vi "A170316-11_Auto - 副本.vi"() -> ()   [LabVIEW 2020]
uses:
  2e0b5f5e-2208-4490-a798-25a802626be8.vi
  Global_Variable/A170316-11.vi
  Global_Variable/Global.vi
  Database/Global1.vi
  <vilib>/addons/database/Connection.llb/DB Tools Open Connec (String).vi
  <vilib>/regexp/Match Regular Expression.xnode
  <vilib>/addons/database/NI_Database_API.lvlib
panel:
  out "请拾取O型圈":bool
  out "请拾取弹簧":bool
  in  "控制器支架":T1(ring)
  in  "ECU步骤":T2(ring)
  in  "电机步骤":T3(ring)
  out "产品型号":string
  in  "更换产品":refnum<vi>
  in  "前序OK？_ECU":string
  in  "前序OK？":string
  in  "Process":string[](array[string])
  in  "Code":string[](array[string])
  in  "User":string[](array[string])
  in  "Result":string[](array[string])
  in  "Device":string[](array[string])
  out "安装支架螺栓4拧紧确认":bool
  in  "STEP2":string
  in  "STEP1":string
  out "控制器安装螺栓3拧紧确认":bool
  out "电机安装螺栓3扭矩确认":bool
  out "控制器支架螺栓5拧紧确认":bool
  out "安装扎带并取走工件":bool
  out "涂色标":bool
  out "按启动按钮拍照确认":bool
  out "电机安装螺栓2扭矩确认":bool
  out "电机安装螺栓1扭矩确认":bool
  out "安装支架涂色标":bool
  out "控制器安装螺栓2拧紧确认":bool
  out "控制器安装螺栓1拧紧确认":bool
  out "安装支架螺栓2拧紧确认":bool
  out "安装弹性垫圈弹簧并按启动拍照":bool
  out "安装支架螺栓1拧紧确认":bool
  out "控制器支架涂色标":bool
  out "控制器支架螺栓4拧紧确认":bool
  out "控制器支架螺栓3拧紧确认":bool
  out "控制器支架螺栓2拧紧确认":bool
  out "控制器支架螺栓1拧紧确认":bool
  out "安装支架螺栓3拧紧确认":bool
  in  "更换布局":string
  out "安装扎带和线卡并取走工件":bool
  out "安装支架扎带安装":bool
  out "安装支架线卡扎带安装":bool
  out "控制器支架安装线卡扎带":bool
  out "磨合次数":i32
  in  "判定结果":bool[][](array[boolean])=[[TRUE]]
  in  "STEP3":string
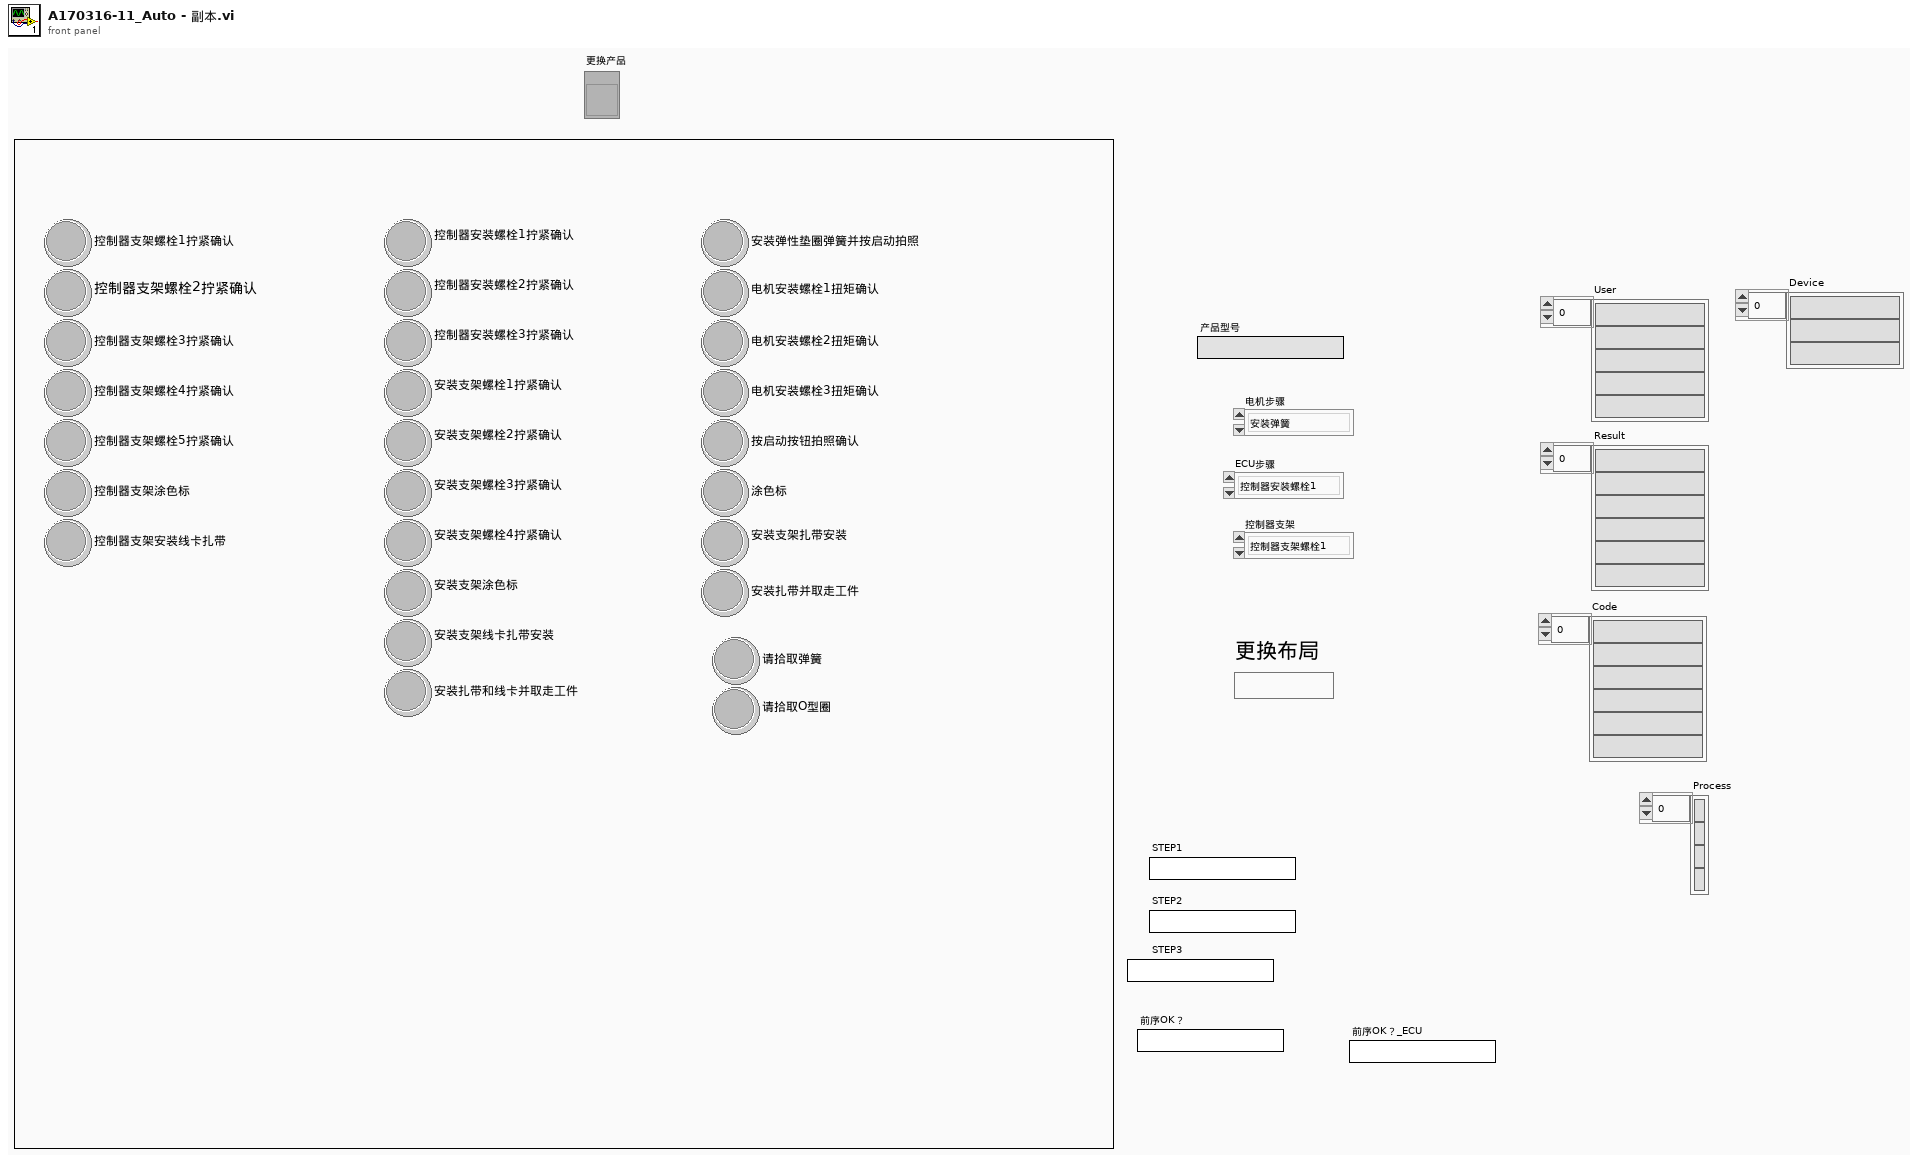
[diagram p1: front panel]
types:
  T1 = enum16{"控制器支架螺栓1", "控制器支架螺栓2", "控制器支架螺栓3", "控制器支架螺栓4", "控制器支架螺栓5", "涂色标", "安装线卡轧带", "完成"}
  T2 = enum16{"控制器安装螺栓1", "控制器安装螺栓2", "控制器安装螺栓3", "安装支架螺栓1", "安装支架螺栓2", "安装支架螺栓3", "安装支架螺栓4", "涂色标", "安装线卡轧带", "取走工件", "完成"}
  T3 = enum16{"安装弹簧", "安装O型圈", "安装弹性垫圈", "电机螺栓1", "电机螺栓2", "电机螺栓3", "电机拍照", "涂色标", "装轧带", "取走工件", "完成"}
  T4 = cluster{i64, i64, i64, "电机工位生产结果":string, "result string":string}
  T5 = cluster{i64, i64, i64, "电机工位生产结果":string, "result string":string}[]
  T6 = typedef "NI_Database_API.lvlib/Conn ObjectReference.ctl" = refnum<k1>
  T7 = cluster{"电机工位生产结果":string, "result string":string}
  T8 = cluster{i64, i64, i64, "ECU工位生产结果":string, "result string":string}
  T9 = cluster{i64, i64, i64, "ECU工位生产结果":string, "result string":string}[]
  T10 = cluster{"ECU工位生产结果":string, "result string":string}
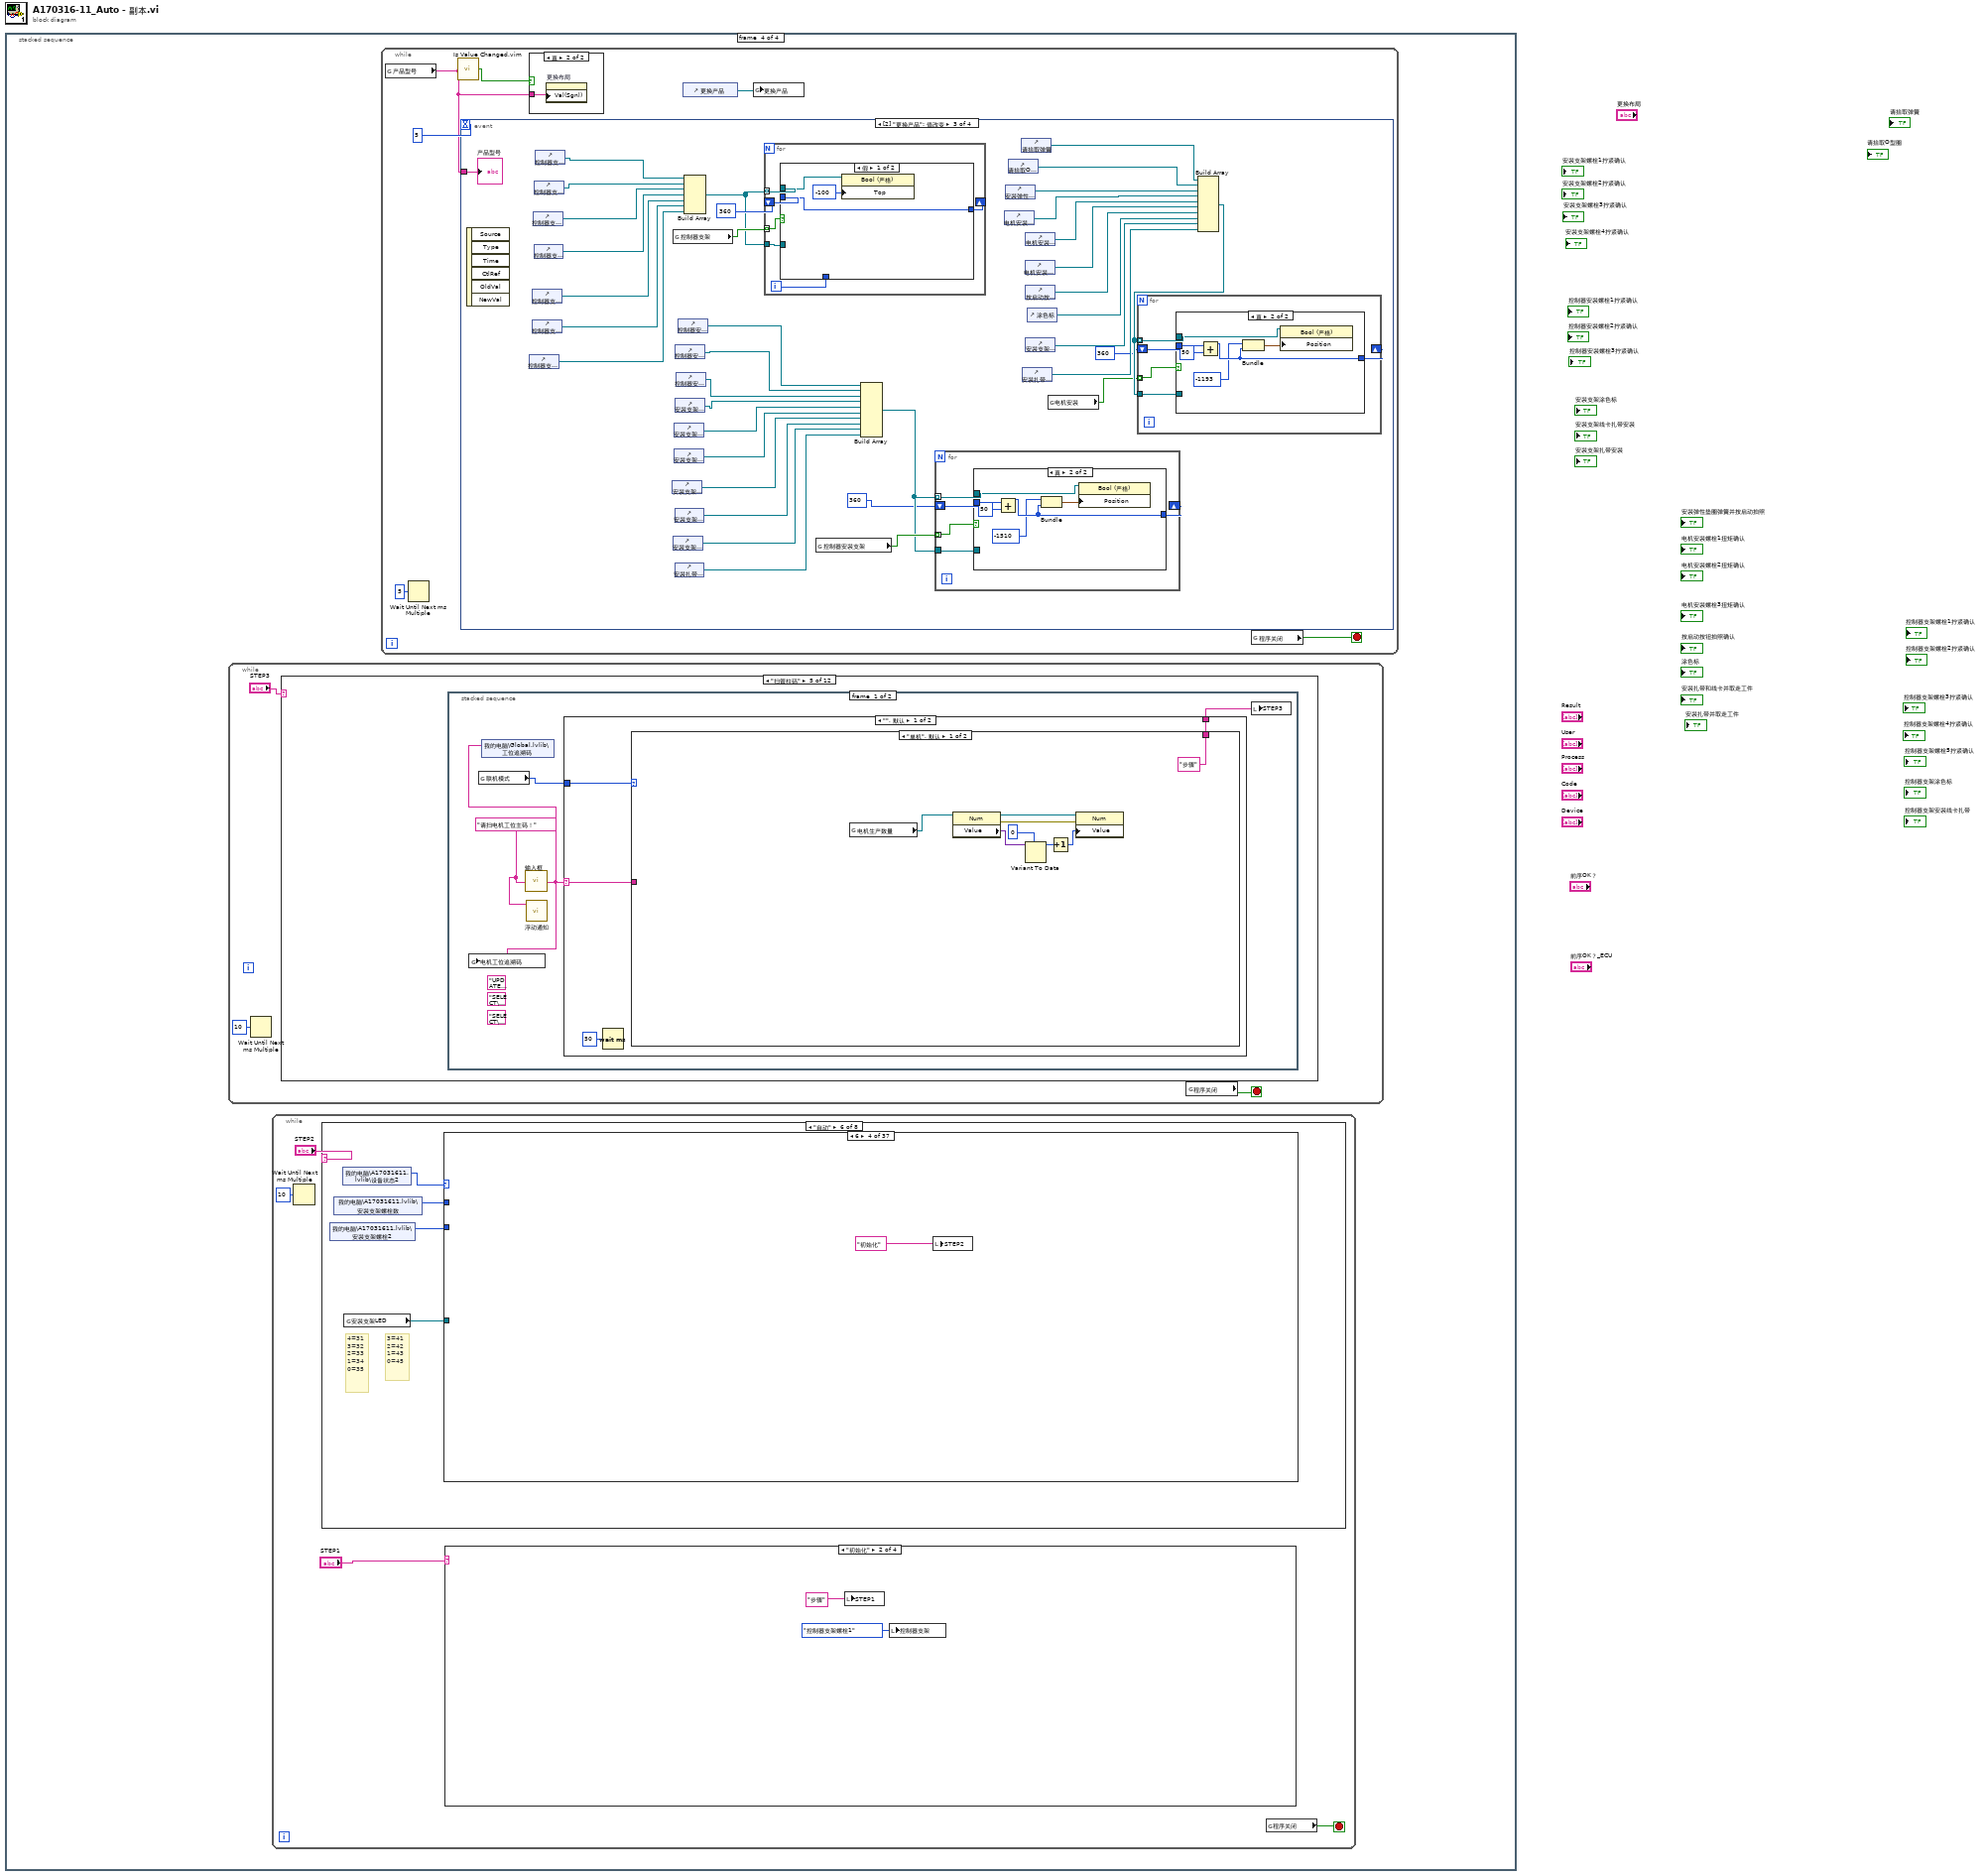
[diagram p0: block diagram]
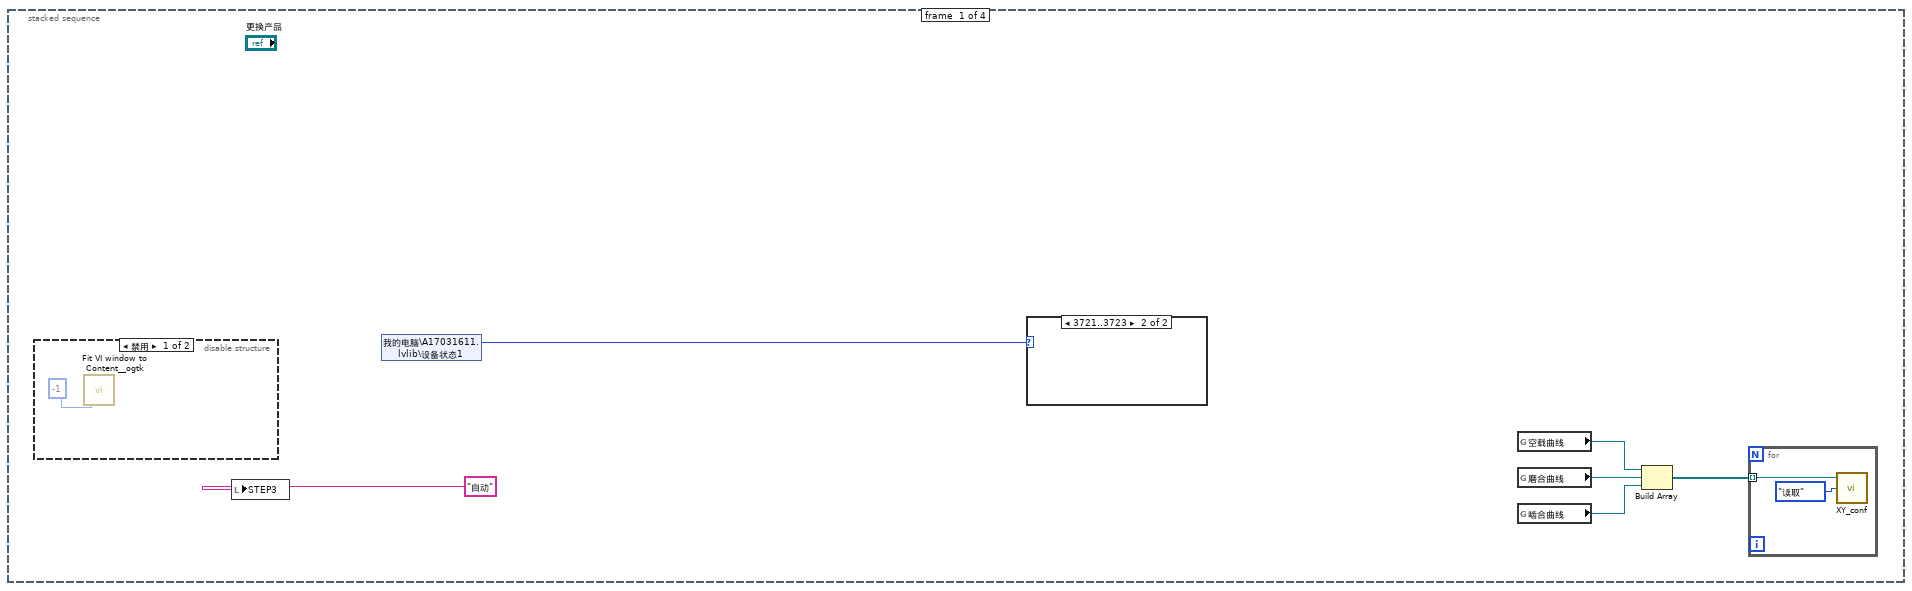
[diagram p2: hidden frame]
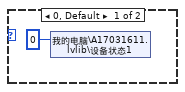
[diagram p4: hidden frame]
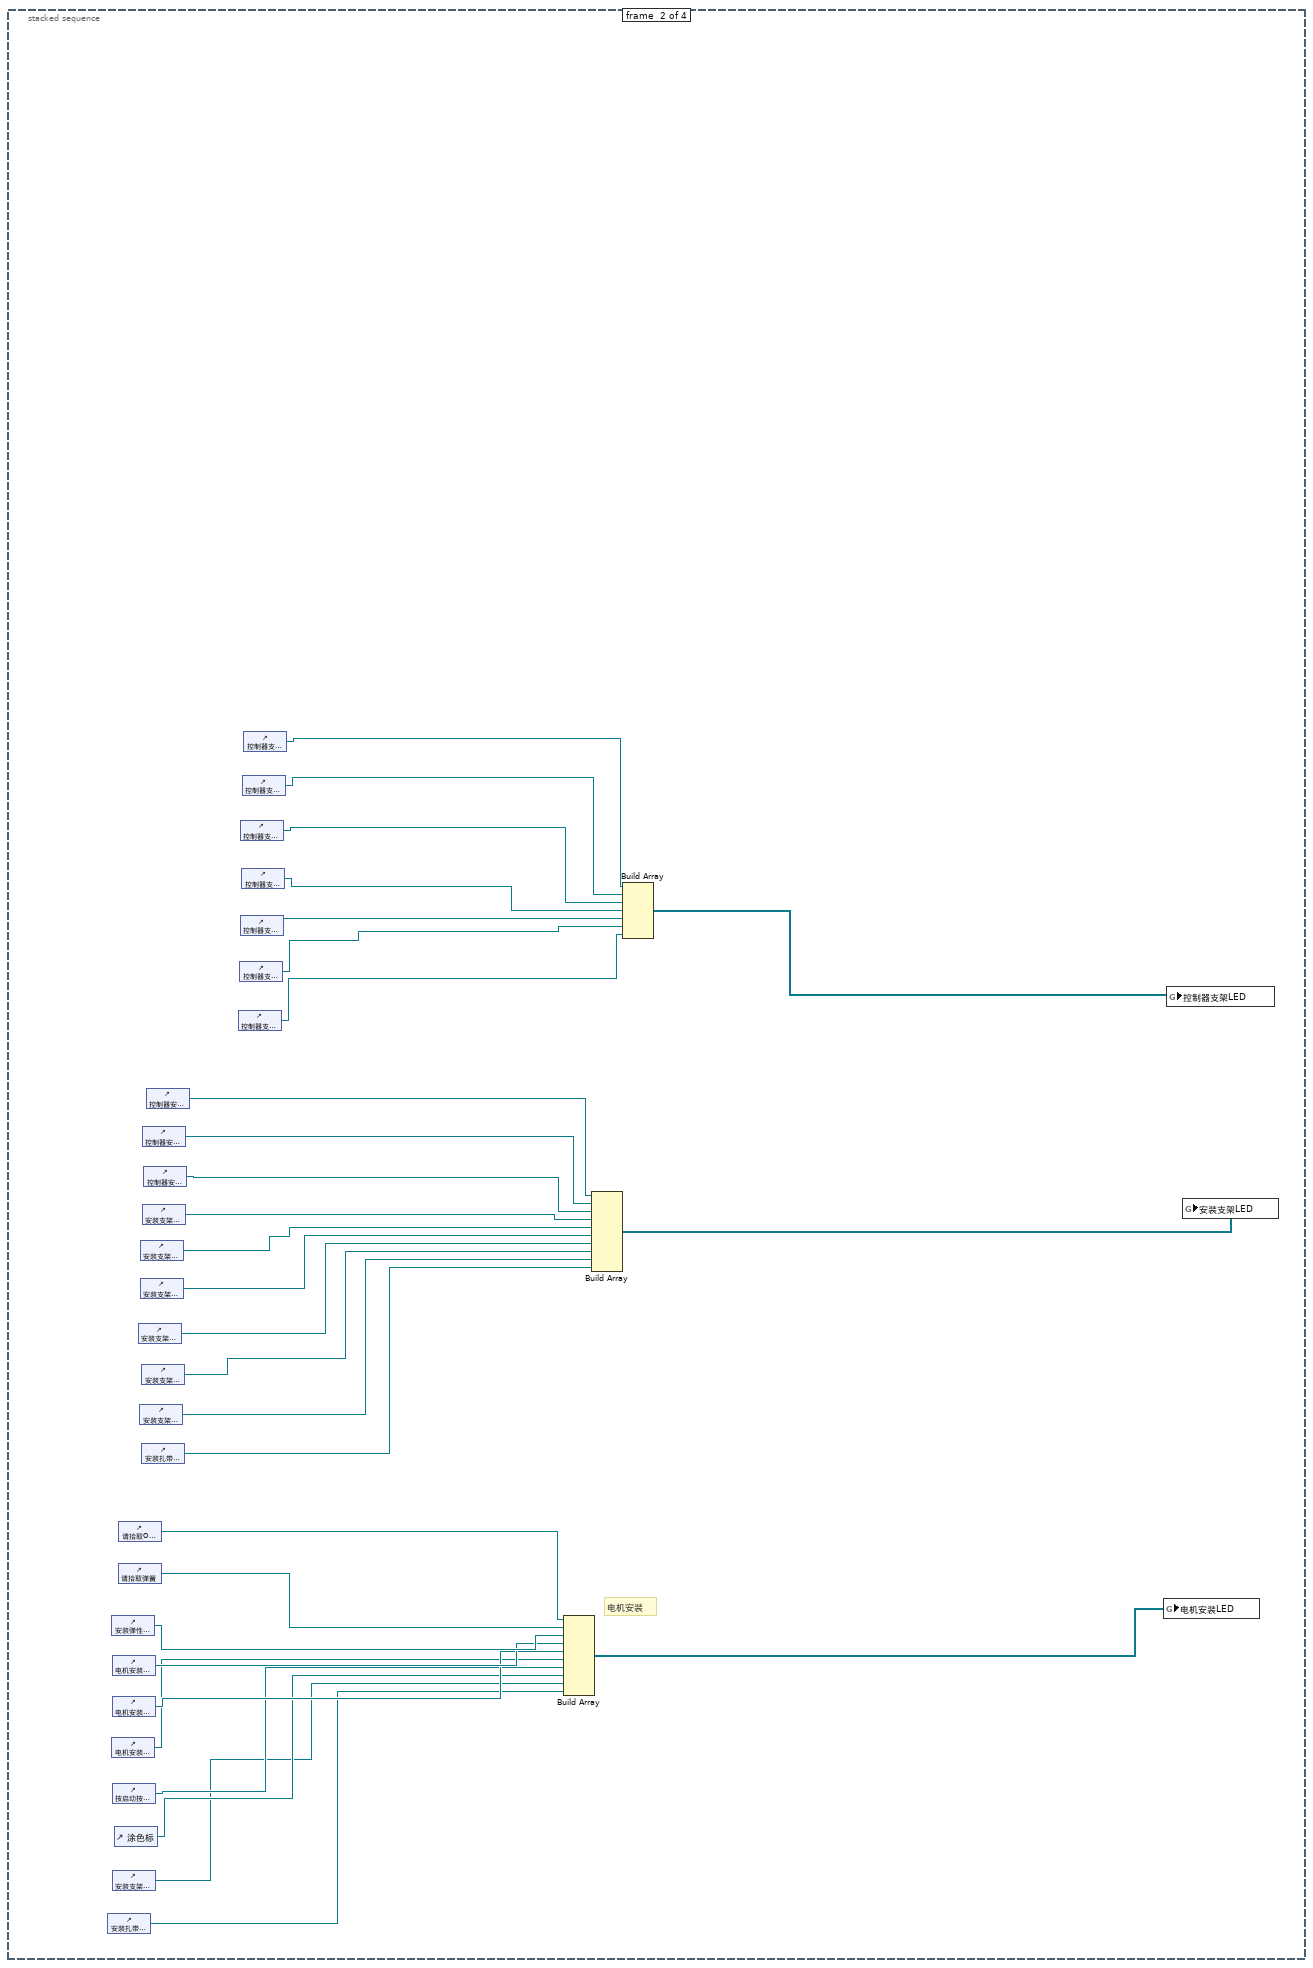
[diagram p5: hidden frame]
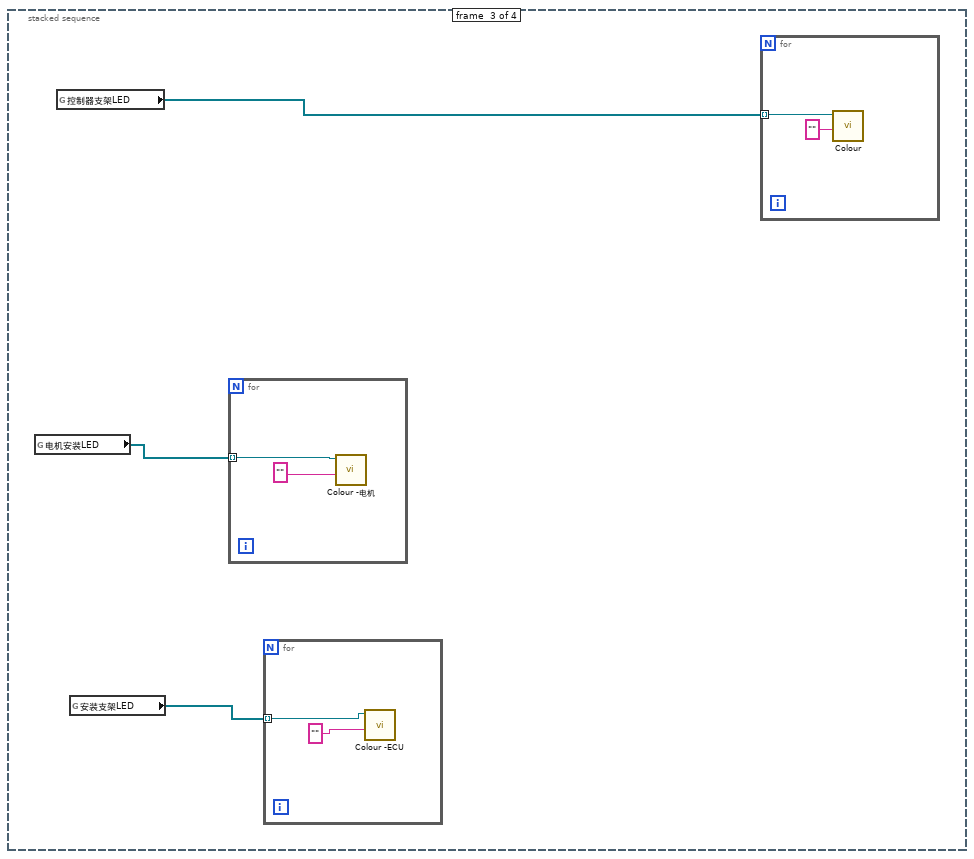
[diagram p6: hidden frame]
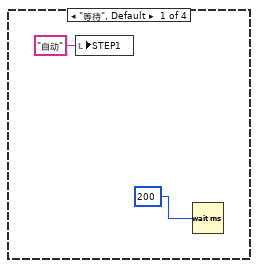
[diagram p7: hidden frame]
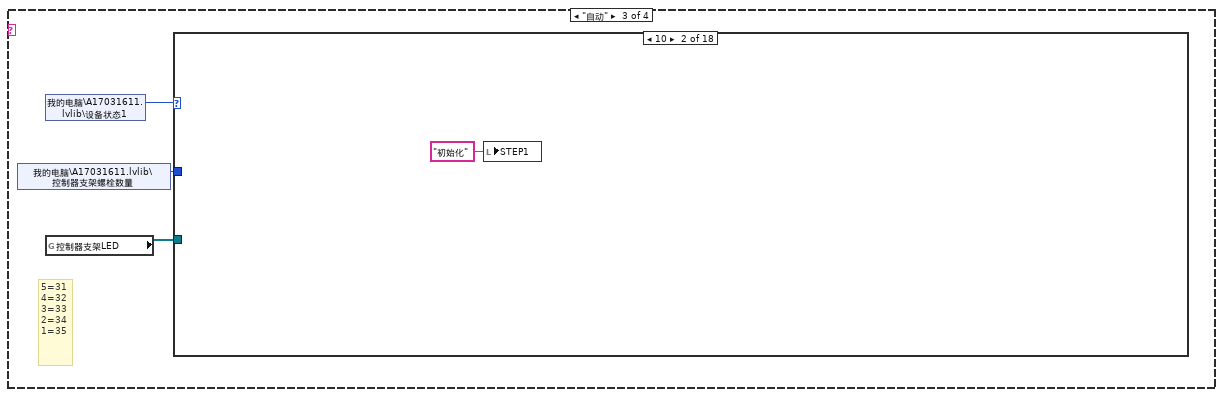
[diagram p8: hidden frame]
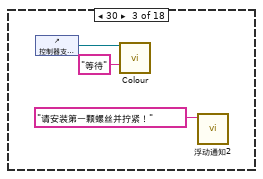
[diagram p10: hidden frame]
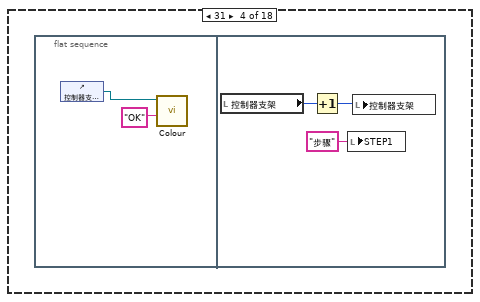
[diagram p11: hidden frame]
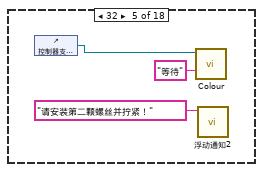
[diagram p12: hidden frame]
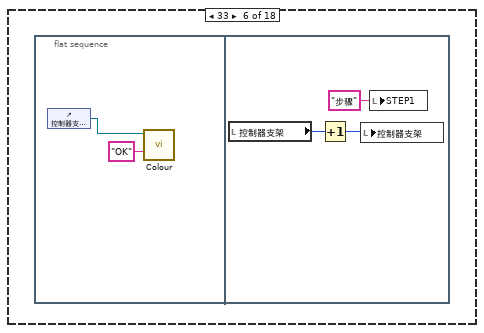
[diagram p13: hidden frame]
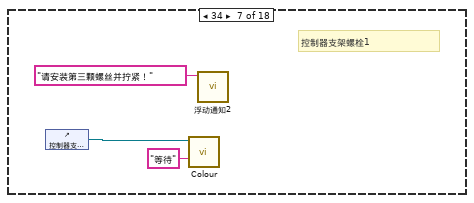
[diagram p14: hidden frame]
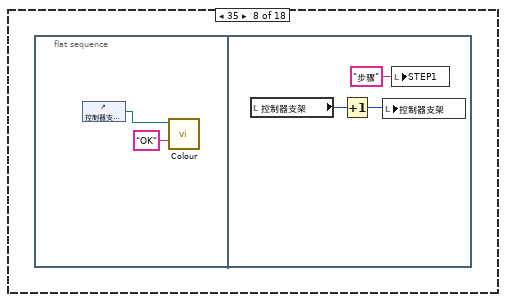
[diagram p15: hidden frame]
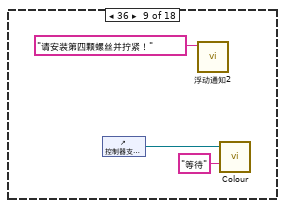
[diagram p16: hidden frame]
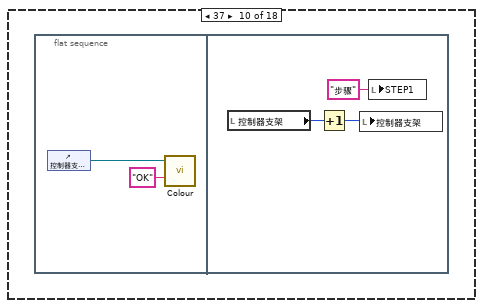
[diagram p17: hidden frame]
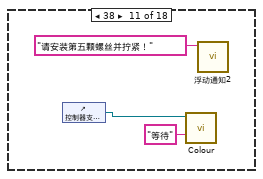
[diagram p18: hidden frame]
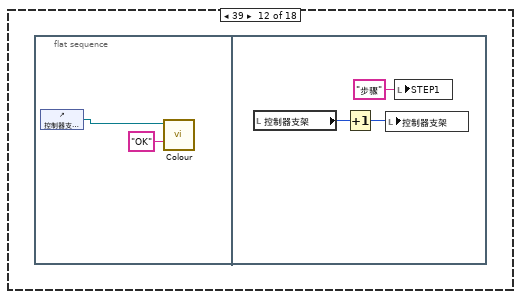
[diagram p19: hidden frame]
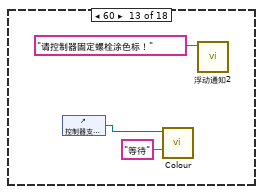
[diagram p20: hidden frame]
diagram:
  n1 = stacked-sequence {
    frame #0 {
      n2 = disable-structure shown="禁用" {
        frame Disabled {
          n3 = call "Fit VI window to Content__ogtk.vi"("border spacing (2 px)"=-1) -> ()  [unwired: 5 in, 2 out]
        }
        frame Enabled {
        }
      }
      n4 = local write "STEP3"("自动" ("STEP")) -> ()
      n5 = shared-variable "我的电脑\\A17031611.lvlib\\设备状态1"() -> (w4:i16)  [unwired: 1 in, 1 out]
      n6 = case shown="3721..3723" w4 {
        frame 0, Default {
          n7 = shared-variable "我的电脑\\A17031611.lvlib\\设备状态1"(i16 0 ("设备状态")) -> ()  [unwired: 1 in, 1 out]
        }
        frame 3721..3723 {
        }
      }
      n8 = global read "A170316-11.vi" "空载曲线"() -> (w1:refnum<vi>)
      n9 = global read "A170316-11.vi" "磨合曲线"() -> (w2:refnum<vi>)
      n10 = global read "A170316-11.vi" "啮合曲线"() -> (w3:refnum<vi>)
      n11 = Build Array(w1, w2, w3) -> (w5:refnum<vi>[])
      n12 = for {
        tunnel: w5 -> [w10] mode=indexing
        n13 = call "XY_conf.vi"("方式"=enum16{"写入", "读取"}."读取", "XY图引用"=w10) -> ()  [unwired: 3 in, 1 out]
      }
    }
    frame #1 {
      # "电机安装"
      n14 = control-ref of="安装扎带并取走工件"() -> (w23:refnum<vi>)
      n15 = control-ref of="安装弹性垫圈弹簧并按启动拍照"() -> (w30:refnum<vi>)
      n16 = control-ref of="电机安装螺栓3扭矩确认"() -> (w27:refnum<vi>)
      n17 = control-ref of="电机安装螺栓1扭矩确认"() -> (w29:refnum<vi>)
      n18 = control-ref of="电机安装螺栓2扭矩确认"() -> (w28:refnum<vi>)
      n19 = control-ref of="按启动按钮拍照确认"() -> (w26:refnum<vi>)
      n20 = control-ref of="安装支架扎带安装"() -> (w24:refnum<vi>)
      n21 = control-ref of="涂色标"() -> (w25:refnum<vi>)
      n22 = control-ref of="请拾取O型圈"() -> (w11:refnum<vi>)
      n23 = control-ref of="请拾取弹簧"() -> (w12:refnum<vi>)
      n24 = control-ref of="安装支架螺栓4拧紧确认"() -> (w16:refnum<vi>)
      n25 = control-ref of="安装支架线卡扎带安装"() -> (w14:refnum<vi>)
      n26 = control-ref of="安装支架螺栓2拧紧确认"() -> (w18:refnum<vi>)
      n27 = control-ref of="安装支架螺栓3拧紧确认"() -> (w17:refnum<vi>)
      n28 = control-ref of="安装支架涂色标"() -> (w15:refnum<vi>)
      n29 = control-ref of="安装扎带和线卡并取走工件"() -> (w13:refnum<vi>)
      n30 = control-ref of="控制器安装螺栓2拧紧确认"() -> (w21:refnum<vi>)
      n31 = control-ref of="安装支架螺栓1拧紧确认"() -> (w19:refnum<vi>)
      n32 = control-ref of="控制器安装螺栓3拧紧确认"() -> (w20:refnum<vi>)
      n33 = control-ref of="控制器安装螺栓1拧紧确认"() -> (w22:refnum<vi>)
      n34 = control-ref of="控制器支架安装线卡扎带"() -> (w31:refnum<vi>)
      n35 = control-ref of="控制器支架涂色标"() -> (w32:refnum<vi>)
      n36 = control-ref of="控制器支架螺栓3拧紧确认"() -> (w35:refnum<vi>)
      n37 = control-ref of="控制器支架螺栓5拧紧确认"() -> (w33:refnum<vi>)
      n38 = control-ref of="控制器支架螺栓4拧紧确认"() -> (w34:refnum<vi>)
      n39 = control-ref of="控制器支架螺栓2拧紧确认"() -> (w36:refnum<vi>)
      n40 = control-ref of="控制器支架螺栓1拧紧确认"() -> (w37:refnum<vi>)
      n41 = Build Array(w11, w12, w30, w29, w28, w27, w26, w25, w24, w23) -> (w40:refnum<vi>[])
      n42 = Build Array(w22, w21, w20, w19, w18, w17, w16, w15, w14, w13) -> (w39:refnum<vi>[])
      n43 = Build Array(w37, w36, w35, w34, w33, w32, w31) -> (w38:refnum<vi>[])
      n44 = global write "A170316-11.vi" "电机安装LED"(w40) -> ()
      n45 = global write "A170316-11.vi" "控制器支架LED"(w38) -> ()
      n46 = global write "A170316-11.vi" "安装支架LED"(w39) -> ()
    }
    frame #2 {
      n47 = global read "A170316-11.vi" "电机安装LED"() -> (w42:refnum<vi>[])
      n48 = global read "A170316-11.vi" "控制器支架LED"() -> (w43:refnum<vi>[])
      n49 = global read "A170316-11.vi" "安装支架LED"() -> (w41:refnum<vi>[])
      n50 = for {
        tunnel: w42 -> [w47] mode=indexing
        n51 = call "Colour -电机.vi"("result"="", "colourRef"=w47) -> ()  [unwired: 9 in, 1 out]
      }
      n52 = for {
        tunnel: w41 -> [w45] mode=indexing
        n53 = call "Colour -ECU.vi"("result"="", "colourRef"=w45) -> ()  [unwired: 9 in, 1 out]
      }
      n54 = for {
        tunnel: w43 -> [w48] mode=indexing
        n55 = call "Colour.vi"("result"="", "colourRef"=w48) -> ()  [unwired: 9 in, 1 out]
      }
    }
    frame #3 {
      n56 = while {
        stop <- w633 stop-if-true
        n57 = Wait Until Next ms Multiple(millisecond multiple=u32 10 ("毫秒倍数")) -> ()  [unwired: 1 out]
        n58 = case shown="\"扫管柱码\"" "STEP3" {
          frame "等待", Default {
            n59 = local write "STEP3"("自动" ("STEP")) -> ()
            n60 = Wait (ms)(milliseconds to wait=u32 100 ("等待时间（毫秒）")) -> ()  [unwired: 1 out]
          }
          frame "手动" {
            n61 = global read "Global.vi" "ECU自动"() -> (w642:refnum<vi>)
            n62 = shared-variable "我的电脑\\A17031611.lvlib\\设备状态1"(u16 0 ("设备状态")) -> ()  [unwired: 1 in, 1 out]
            n63 = shared-variable "我的电脑\\A17031611.lvlib\\设备状态2"(u16 0 ("设备状态")) -> ()  [unwired: 1 in, 1 out]
            n64 = property class="Bool (严格)"(reference=w642, "Value"=FALSE) -> ()  [unwired: 1 in, 2 out]
            n65 = local write "STEP2"("等待" ("STEP")) -> ()
            n66 = local write "STEP1"("等待" ("STEP1")) -> ()
            n67 = global read "Global.vi" "电机程序自动"() -> (w645:refnum<vi>)
            n68 = shared-variable "我的电脑\\A17031611.lvlib\\设备状态3"(u16 0 ("设备状态")) -> ()  [unwired: 1 in, 1 out]
            n69 = property class="Bool"(reference=w645, "Value"=FALSE) -> ()  [unwired: 1 in, 2 out]
            n70 = local write "STEP3"("等待" ("STEP")) -> ()
            n71 = Wait (ms)(milliseconds to wait=u32 100 ("等待时间（毫秒）")) -> ()  [unwired: 1 out]
          }
          frame "初始化" {
            n72 = stacked-sequence {
              frame #0 {
                w657 = enum16{"录入", "清空"}."清空" ("功能")
                n73 = global read "Global.vi" "电机生产数量"() -> (w650:refnum<vi>)
                n74 = shared-variable "我的电脑\\Global.lvlib\\工位追溯码"("" ("传感器码")) -> ()  [unwired: 1 in, 1 out]
                n75 = call "物料信息录入.vi"("功能"=w657) -> ("错误输出"=w656:errorcluster)  [unwired: 14 in]
                n76 = call "质量信息录入.vi"("功能"=w657, "错误输入（无错误）"=w656) -> ("错误输出"=w658:errorcluster)  [unwired: 13 in]
                n77 = property class="Num"(reference=w650, "Value"=0 ("磨合次数")) -> ()  [unwired: 1 in, 2 out]
                n78 = call "不合格信息录入.vi"("功能"=w657, "错误输入（无错误）"=w658) -> ()  [unwired: 13 in, 1 out]
                n79 = global read "Global.vi" "电机程序自动"() -> (w654:refnum<vi>)
                n80 = global read "Global.vi" "检测结果"() -> (w652:refnum<vi>)
                n81 = shared-variable "我的电脑\\A17031611.lvlib\\设备状态3"(i16 6 ("设备状态")) -> ()  [unwired: 1 in, 1 out]
                n82 = property class="Bool"(reference=w654, "Value"=TRUE) -> ()  [unwired: 1 in, 2 out]
                n83 = call "Colour.vi"("result"="", "colourRef"=w652) -> ()  [unwired: 9 in, 1 out]
              }
              frame #1 {
                n84 = for {
                  N: 2 -> [_]
                  tunnel: [cluster{dbl[], dbl[]} {[], []}] -> _ mode=indexing
                }
              }
              frame #2 {
                n85 = global read "Global.vi" "Result"() -> (w663:refnum<vi>)
                n86 = property class="Tbl"(reference=w663, "Value"=string[][] []) -> (reference out=w664:refnum<vi>, error out=w665:errorcluster)  [unwired: 1 in]
                n87 = property class="Tbl"(reference=w664, error in=w665, "Row Headers[]"=string[] ["正向空载扭矩最大值", "正向空载扭矩最小值", "正向空载扭矩平均值", "正向空载扭矩波动值", "逆向空载扭矩最大值", "逆向空载扭矩最小值", "逆向空载扭矩平均值", "逆向空载扭矩波动值", "啮合间隙"] ("列首字符串[]")) -> ()  [unwired: 2 out]
              }
              frame #3 {
                n88 = local write "电机步骤"(T3."安装弹簧" ("电机步骤")) -> ()
                n89 = local write "STEP3"("等待" ("STEP")) -> ()
              }
            }
          }
          frame "批次数量判断" {
            n90 = shared-variable "我的电脑\\Global.lvlib\\产品型号"() -> (w673:string, error out=w676:errorcluster)  [unwired: 1 in]
            n91 = global read "Global.vi" "批次"() -> (w674:refnum<vi>)
            n92 = call "获取批次信息.vi"("error in (no error)"=w676, "产品型号"=w673, "Tbl引用句柄"=w674) -> ("error out"=w675:errorcluster)  [unwired: 7 in, 1 out]
            n93 = property class="Tbl"(reference=w674, error in=w675) -> ("Value"=w677:string[][])  [unwired: 2 out]
            n94 = for {
              tunnel: w677 -> [w683] mode=indexing
              tunnel: [w678] -> w672 mode=indexing
              n95 = Index Array(array=w683) -> (element #1=w679:string, element #3=w682:string)  [unwired: 3 in, 1 out]
              n96 = Decimal String To Number(string=w682) -> (number=w681:i32)  [unwired: 2 in, 1 out]
              n97 = Less Or Equal To 0?(x=w681) -> (x <= 0?=w680:bool)
              n98 = case shown="真" w680 {
                tunnel: w679 -> [_ w688]
                tunnel: [TRUE FALSE] -> w678
                frame False {
                }
                frame True {
                  n99 = Concatenate Strings(w688, "数量不足！" ("字符串")) -> (w686:string)
                  n100 = One Button Dialog(message=w686) -> ()  [unwired: 1 in, 1 out]
                }
              }
            }
            n101 = And Array Elements(Boolean array=w672) -> (logical AND=w671:bool)
            n102 = Select(t="扫码" ("STEP"), s=w671, f="手动" ("STEP")) -> (s? t:f=w668:string)
            n103 = local write "STEP3"(w668) -> ()
          }
          frame "扫管柱码" {
            n104 = stacked-sequence {
              frame #0 {
                (unwired) "SELECT\ndbo.[Code].CODE_ID,\ndbo.[Code].CODE_MAIN,\ndbo.[Code].PRODUCT_ID\n\nFROM\ndbo.[Code].CODE_MAIN = 'MACAU3001'" ("格式字符串")
                (unwired) "SELECT\n*\nFROM\ndbo.[Code]\nWHERE\ndbo.[Code].CODE_MAIN = 'MACAU3001'" ("格式字符串")
                (unwired) "UPDATE\ndbo.[Code]\nSET dbo.[Code].CODE_SENSOR = 'henglong'\nWHERE\ndbo.[Code].CODE_MAIN = 'MACAU3001'\n" ("格式字符串")
                w689 = "请扫电机工位主码！" ("提示信息")
                n105 = global read "Global1.vi" "联机模式"() -> (w691:enum16{"单机", "联网"})
                n106 = call "输入框.vi"("提示信息"=w689) -> ("条形码输出"=w690:string)
                n107 = global write "Global1.vi" "电机工位追溯码"(w690) -> ()
                n108 = shared-variable "我的电脑\\Global.lvlib\\工位追溯码"(w690) -> ()  [unwired: 1 in, 1 out]
                n109 = call "浮动通知.vi"("通知内容"=w689) -> ()  [unwired: 11 in]
                n110 = case shown="\"\", 默认" w690 {
                  selector: w690 -> [w695 _]
                  tunnel: [w694 "手动"] -> w692
                  tunnel: w691 -> [w693 _]
                  frame "", Default {
                    n111 = Wait (ms)(milliseconds to wait=u32 50 ("等待时间（毫秒）")) -> ()  [unwired: 1 out]
                    n112 = case shown="\"单机\", 默认" w693 {
                      tunnel: w695 -> [_ w706]
                      tunnel: ["步骤" ("State(s) in Front (\"\")") w705] -> w694
                      frame "单机", Default {
                        n113 = global read "Global.vi" "电机生产数量"() -> (w699:refnum<vi>)
                        n114 = property class="Num"(reference=w699) -> (reference out=w697:refnum<vi>, error out=w701:errorcluster, "Value"=w702:variant)  [unwired: 1 in]
                        n115 = Variant To Data(type=u32 0, Variant=w702) -> (data=w703:u32)  [unwired: 1 in, 1 out]
                        n116 = Increment(x=w703) -> (x+1=w704:u32)
                        n117 = property class="Num"(reference=w697, error in=w701, "Value"=w704) -> ()  [unwired: 2 out]
                      }
                      frame "联网" {
                        n118 = stacked-sequence {
                          tunnel: w706 -> [w713 _ _ _]
                          tunnel: [_ _ _ w735] -> w705
                          frame #0 {
                            n119 = global read "Global1.vi" "PRODUCT_ID"() -> (w710:string)
                            n120 = Format Into String(format string="SELECT\ndbo.[Code].CODE_ID\nFROM\ndbo.[Code]\nWHERE\ndbo.[Code].CODE_MAIN = '%s'\nAND\ndbo.[Code].PRODUCT_ID = %s\n" ("格式字符串"), w713, w710) -> (resulting string=w712:string)  [unwired: 2 in, 1 out]
                            n121 = call "SQL_query.vi"("SQL query"=w712, "联机模式"=enum16{"单机", "联网"}."联网") -> ("data"=w716:string[][])  [unwired: 1 in, 2 out]
                            n122 = Index Array(array=w716, index (row)=0 ("索引 (行)")) -> (element=w715:string[])  [unwired: 1 in]
                            n123 = Index Array(array=w715, index=0 ("索引")) -> (element=w707:string)
                            n124 = global write "Global1.vi" "CODE_ID"(w707) -> ()
                          }
                          frame #1 {
                            n125 = global read "Global1.vi" "前序DEVICE_ID"() -> (w717:string)
                            n126 = global read "Global1.vi" "CODE_ID"() -> (w718:string)
                            n127 = Format Into String(format string="SELECT\ndbo.[Result].RESULT_VALUE\nFROM\ndbo.[Result]\nWHERE\ndbo.[Result].DEVICE_ID = '%s'\nAND\ndbo.[Result].CODE_ID = %s\n" ("格式字符串"), w717, w718) -> (resulting string=w723:string)  [unwired: 2 in, 1 out]
                            n128 = call "SQL_query.vi"("SQL query"=w723, "联机模式"=enum16{"单机", "联网"}."联网") -> ("data"=w726:string[][])  [unwired: 1 in, 2 out]
                            n129 = Index Array(array=w726, index (row)=0 ("索引 (行)")) -> (element=w725:string[])  [unwired: 1 in]
                            n130 = Index Array(array=w725, index=0 ("索引")) -> (element=w719:string)
                            n131 = local write "前序OK？"(w719) -> ()
                          }
                          frame #2 {
                            n132 = disable-structure shown="禁用" {
                              frame Disabled {
                                n133 = global read "Global1.vi" "CODE_ID"() -> (w728:string)
                                n134 = Format Into String(format string="SELECT\ndbo.[Result].RESULT_VALUE\nFROM\ndbo.[Result]\nWHERE\ndbo.[Result].CODE_ID = '%s''" ("格式字符串"), w728) -> (resulting string=w730:string)  [unwired: 2 in, 1 out]
                                n135 = call "SQL_query.vi"("SQL query"=w730, "联机模式"=enum16{"单机", "联网"}."联网") -> ("data"=w733:string[][])  [unwired: 1 in, 2 out]
                                n136 = Index Array(array=w733) -> (element=w731:string[])  [unwired: 2 in]
                                n137 = Index Array(array=w731) -> (element=w732:string)  [unwired: 1 in]
                                n138 = global write "Global1.vi" "RESULT_VALUE"(w732) -> ()
                              }
                              frame Enabled {
                              }
                            }
                          }
                          frame #3 {
                            n139 = local read "前序OK？"() -> (w734:string)
                            n140 = case shown="\"OK\"" w734 {
                              tunnel: ["等待" "等待" "步骤"] -> w735
                              frame Default {
                                (unwired) i16 6 ("设备状态控制字")
                                n141 = global read "Global1.vi" "电机上序状态"() -> (w739:refnum<vi>)
                                n142 = call "浮动通知.vi"("通知内容"="上序漏序！！" ("Status")) -> ()  [unwired: 11 in]
                                n143 = global read "Global.vi" "电机前序显示字"() -> (w737:refnum<vi>)
                                n144 = call "Colour.vi"("result"="等待", "colourRef"=w739) -> ()  [unwired: 9 in, 1 out]
                                n145 = Wait (ms)(milliseconds to wait=u32 2000 ("等待时间（毫秒）")) -> ()  [unwired: 1 out]
                                n146 = property class="Str"(reference=w737, "Value"="漏序 " ("值")) -> ()  [unwired: 1 in, 2 out]
                              }
                              frame "NG" {
                                (unwired) i16 6 ("设备状态控制字")
                                n147 = global read "Global1.vi" "电机上序状态"() -> (w746:refnum<vi>)
                                n148 = call "浮动通知.vi"("通知内容"="上序生产结果不合格！" ("Status")) -> ()  [unwired: 11 in]
                                n149 = global read "Global.vi" "电机前序显示字"() -> (w744:refnum<vi>)
                                n150 = call "Colour.vi"("result"="NG", "colourRef"=w746) -> ()  [unwired: 9 in, 1 out]
                                n151 = Wait (ms)(milliseconds to wait=u32 2000 ("等待时间（毫秒）")) -> ()  [unwired: 1 out]
                                n152 = property class="Str"(reference=w744, "Value"="NG " ("值")) -> ()  [unwired: 1 in, 2 out]
                              }
                              frame "OK" {
                                n153 = global read "Global.vi" "电机生产数量"() -> (w760:refnum<vi>)
                                n154 = global read "Global1.vi" "电机上序状态"() -> (w753:refnum<vi>)
                                n155 = property class="Num"(reference=w760) -> (reference out=w761:refnum<vi>, error out=w759:errorcluster, "Value"=w758:variant)  [unwired: 1 in]
                                n156 = global read "Global.vi" "电机前序显示字"() -> (w751:refnum<vi>)
                                n157 = call "Colour.vi"("result"="OK", "colourRef"=w753) -> ()  [unwired: 9 in, 1 out]
                                n158 = Variant To Data(type=u32 0, Variant=w758) -> (data=w757:u32)  [unwired: 1 in, 1 out]
                                n159 = Increment(x=w757) -> (x+1=w756:u32)
                                n160 = property class="Num"(reference=w761, error in=w759, "Value"=w756) -> ()  [unwired: 2 out]
                                n161 = property class="Str"(reference=w751, "Value"="OK" ("值")) -> ()  [unwired: 1 in, 2 out]
                              }
                            }
                          }
                        }
                      }
                    }
                  }
                  frame "exit" {
                  }
                }
                n162 = local write "STEP3"(w692) -> ()
              }
              frame #1 {
                n163 = Wait (ms)(milliseconds to wait=u32 100 ("等待时间（毫秒）")) -> ()  [unwired: 1 out]
              }
            }
          }
          frame "扫电机码" {
            n164 = stacked-sequence {
              frame #0 {
                w764 = "请扫电机码！" ("提示信息")
                n165 = call "输入框.vi"("提示信息"=w764) -> ("条形码输出"=w765:string)
                n166 = call "浮动通知.vi"("通知内容"=w764) -> ()  [unwired: 11 in]
                n167 = case shown="\"\", 默认" w765 {
                  selector: w765 -> [w767 _]
                  tunnel: [w768 "手动"] -> w766
                  frame "", Default {
                    n168 = global read "Global1.vi" "联机模式"() -> (w769:enum16{"单机", "联网"})
                    n169 = shared-variable "我的电脑\\Global.lvlib\\电机码"(w767) -> ()  [unwired: 1 in, 1 out]
                    n170 = global write "Global1.vi" "电机码"(w767) -> ()
                    n171 = case shown="\"联网\"" w769 {
                      tunnel: w767 -> [_ _]
                      tunnel: ["等待" ("State(s) in Front (\"\")") "等待" ("State(s) in Front (\"\")")] -> w768
                      frame "单机", Default {
                        n172 = shared-variable "我的电脑\\A17031611.lvlib\\设备状态3"(i16 40 ("设备状态控制字")) -> ()  [unwired: 1 in, 1 out]
                      }
                      frame "联网" {
                        n173 = disable-structure shown="禁用" {
                          frame Disabled {
                            n174 = shared-variable "我的电脑\\A17031611.lvlib\\电机安装螺栓数量"() -> (w774:i16)  [unwired: 1 in, 1 out]
                            n175 = case shown="2, 默认" w774 {
                              frame 2, Default {
                                n176 = shared-variable "我的电脑\\A17031611.lvlib\\设备状态3"(i16 41 ("设备状态控制字")) -> ()  [unwired: 1 in, 1 out]
                              }
                              frame 3 {
                                n177 = shared-variable "我的电脑\\A17031611.lvlib\\设备状态3"(i16 40 ("设备状态控制字")) -> ()  [unwired: 1 in, 1 out]
                              }
                            }
                          }
                          frame Enabled {
                          }
                        }
                        n178 = shared-variable "我的电脑\\A17031611.lvlib\\设备状态3"(i16 40 ("设备状态控制字")) -> ()  [unwired: 1 in, 1 out]
                      }
                    }
                  }
                  frame "exit" {
                  }
                }
                n179 = local write "STEP3"(w766) -> ()
              }
              frame #1 {
                n180 = Wait (ms)(milliseconds to wait=u32 100 ("等待时间（毫秒）")) -> ()  [unwired: 1 out]
              }
            }
          }
          frame "录入批次" {
            n181 = shared-variable "我的电脑\\Global.lvlib\\产品型号"() -> (w780:string)  [unwired: 1 in, 1 out]
            n182 = call "更新批次.vi"("型号"=w780) -> ("error out"=w781:errorcluster)  [unwired: 10 in]
            n183 = call "更新易损件.vi"("error in (no error)"=w781) -> ("error out"=w784:errorcluster)  [unwired: 10 in]
            n184 = global read "Global.vi" "批次"() -> (w782:refnum<vi>)
            n185 = property class="Tbl"(reference=w782, error in=w784) -> ("Value"=w783:string[][])  [unwired: 2 out]
            n186 = for {
              tunnel: w783 -> [w787] mode=indexing
              n187 = Index Array(array=w787) -> (element #1=w786:string, element #2=w785:string)  [unwired: 2 in]
              n188 = call "物料信息录入.vi"("物料名称"=w786, "功能"=enum16{"录入", "清空"}."录入", "物料编码"=w785) -> ()  [unwired: 12 in, 1 out]
            }
            n189 = local write "STEP3"("等待" ("STEP")) -> ()
          }
          frame "自动" {
            n190 = shared-variable "我的电脑\\A17031611.lvlib\\电机安装螺栓数量"() -> (w789:i16)  [unwired: 1 in, 1 out]
            n191 = shared-variable "我的电脑\\A17031611.lvlib\\设备状态3"() -> (w790:i16)  [unwired: 1 in, 1 out]
            n192 = global read "A170316-11.vi" "电机安装LED"() -> (w791:refnum<vi>[])
            n193 = case shown="7" w790 {
              tunnel: w789 -> [_ _ _ _ _ _ _ _ _ _ _ _ _ _ _ w844 w855 _ _ _ _ _ _ w908 w920 _ _ _ _ _ _ _ _ _ _ _ _ _ _ _]
              tunnel: w791 -> [_ _ _ _ w796 _ _ _ _ _ _ _ _ w830 w835 w846 w854 _ _ _ _ _ _ w907 w919 w934 _ _ w947 _ w957 w960 _ _ w1003 _ _ _ _ _]
              frame -128 {
                n194 = call "浮动通知.vi"("通知内容"="复位中……" ("Status")) -> ()  [unwired: 11 in]
                n195 = global read "Global.vi" "电机程序自动"() -> (w793:refnum<vi>)
                n196 = property class="Bool"(reference=w793, "Value"=FALSE) -> ()  [unwired: 1 in, 2 out]
              }
              frame 0 {
              }
              frame 5 {
                n197 = call "浮动通知.vi"("通知内容"="复位完成" ("Status")) -> ()  [unwired: 11 in]
              }
              frame 6 {
              }
              frame 7 {
                n198 = for {
                  tunnel: w796 -> [w804] mode=indexing
                  n199 = call "Colour -电机.vi"("result"="", "colourRef"=w804) -> ()  [unwired: 9 in, 1 out]
                }
                n200 = global read "Global.vi" "电机结果显示"() -> (w800:refnum<vi>)
                n201 = shared-variable "我的电脑\\Global.lvlib\\工位追溯码"("" ("传感器码")) -> ()  [unwired: 1 in, 1 out]
                n202 = property class="Str"(reference=w800, "Value"="..." ("结果显示")) -> (reference out=w799:refnum<vi>)  [unwired: 1 in, 1 out]
                n203 = property class="Str"(reference=w799, "Text.TextColor"=u32 16776960) -> ()  [unwired: 1 in, 2 out]
                n204 = local write "STEP3"("扫管柱码" ("STEP3")) -> ()
              }
              frame 8 {
                n205 = call "浮动通知.vi"("通知内容"="程序停止！" ("Status")) -> ()  [unwired: 11 in]
              }
              frame 9 {
                n206 = call "浮动通知.vi"("通知内容"="套花键中" ("Status")) -> ()  [unwired: 11 in]
              }
              frame 10 {
                n207 = local write "STEP3"("步骤" ("STEP3")) -> ()
                n208 = call "浮动通知.vi"("通知内容"="请安装胶垫弹簧并拍照确认！" ("Status")) -> ()  [unwired: 11 in]
              }
              frame 20 {
                n209 = control-ref of="安装弹性垫圈弹簧并按启动拍照"() -> (w809:refnum<vi>)
                n210 = call "Colour -电机.vi"("result"="等待", "colourRef"=w809) -> ()  [unwired: 9 in, 1 out]
              }
              frame 16 {
                n211 = call "浮动通知.vi"("通知内容"="请拾取弹簧并安装到位") -> ()  [unwired: 11 in]
                n212 = control-ref of="请拾取弹簧"() -> (w812:refnum<vi>)
                n213 = call "Colour -电机.vi"("result"="等待", "colourRef"=w812) -> ()  [unwired: 9 in, 1 out]
              }
              frame 17 {
                n214 = flat-sequence {
                  frame #0 {
                    n215 = control-ref of="请拾取弹簧"() -> (w814:refnum<vi>)
                    n216 = call "Colour -电机.vi"("result"="OK", "colourRef"=w814) -> ()  [unwired: 9 in, 1 out]
                  }
                  frame #1 {
                    n217 = local read "电机步骤"() -> (w818:T3)
                    n218 = Increment(x=w818) -> (x+1=w817:T3)
                    n219 = local write "STEP3"("步骤" ("STEP3")) -> ()
                    n220 = Wait (ms)(milliseconds to wait=u32 20 ("等待时间（毫秒）")) -> ()  [unwired: 1 out]
                    n221 = local write "电机步骤"(w817) -> ()
                  }
                }
              }
              frame 18 {
                n222 = control-ref of="请拾取O型圈"() -> (w821:refnum<vi>)
                n223 = call "浮动通知.vi"("通知内容"="请拾O型圈") -> ()  [unwired: 11 in]
                n224 = call "Colour -电机.vi"("result"="等待", "colourRef"=w821) -> ()  [unwired: 9 in, 1 out]
              }
              frame 19 {
                n225 = flat-sequence {
                  frame #0 {
                    n226 = control-ref of="请拾取O型圈"() -> (w823:refnum<vi>)
                    n227 = call "Colour -电机.vi"("result"="OK", "colourRef"=w823) -> ()  [unwired: 9 in, 1 out]
                  }
                  frame #1 {
                    n228 = local read "电机步骤"() -> (w827:T3)
                    n229 = Increment(x=w827) -> (x+1=w826:T3)
                    n230 = local write "STEP3"("步骤" ("STEP3")) -> ()
                    n231 = local write "电机步骤"(w826) -> ()
                    n232 = Wait (ms)(milliseconds to wait=u32 20 ("等待时间（毫秒）")) -> ()  [unwired: 1 out]
                  }
                }
              }
              frame 30 {
                n233 = Index Array(array=w830, index #1=0 ("索引")) -> ()  [unwired: 1 in, 2 out]
                n234 = shared-variable "我的电脑\\A17031611.lvlib\\设备状态3"(i16 20 ("设备状态")) -> ()  [unwired: 1 in, 1 out]
                n235 = control-ref of="安装弹性垫圈弹簧并按启动拍照"() -> (w829:refnum<vi>)
                n236 = call "Colour.vi"("result"="NG", "colourRef"=w829) -> ()  [unwired: 9 in, 1 out]
                n237 = call "浮动通知.vi"("通知内容"="请安装胶垫弹簧并拍照确认！" ("Status")) -> ()  [unwired: 11 in]
              }
              frame 31 {
                n238 = Index Array(array=w835, index #1=0 ("索引")) -> ()  [unwired: 1 in, 2 out]
                n239 = flat-sequence {
                  frame #0 {
                    n240 = control-ref of="安装弹性垫圈弹簧并按启动拍照"() -> (w838:refnum<vi>)
                    n241 = call "浮动通知.vi"("通知内容"="请扫电机码！" ("Status")) -> ()  [unwired: 11 in]
                    n242 = call "Colour -电机.vi"("result"="OK", "colourRef"=w838) -> ()  [unwired: 9 in, 1 out]
                  }
                  frame #1 {
                    n243 = local read "电机步骤"() -> (w843:T3)
                    n244 = Increment(x=w843) -> (x+1=w842:T3)
                    n245 = Wait (ms)(milliseconds to wait=u32 20 ("等待时间（毫秒）")) -> ()  [unwired: 1 out]
                    n246 = local write "电机步骤"(w842) -> ()
                    n247 = local write "STEP3"("步骤" ("STEP3")) -> ()
                  }
                }
              }
              frame 35 {
                n248 = case shown="2" w844 {
                  tunnel: w846 -> [_ w852]
                  frame 0, Default {
                  }
                  frame 2 {
                    n249 = Index Array(array=w852, index #1=0 ("索引")) -> (element #1=w850:refnum<vi>, element #2=w848:refnum<vi>)  [unwired: 1 in]
                    n250 = call "Colour -电机.vi"("result"="OK", "colourRef"=w850) -> ()  [unwired: 9 in, 1 out]
                    n251 = call "Colour -电机.vi"("result"="等待", "colourRef"=w848) -> ()  [unwired: 9 in, 1 out]
                    n252 = shared-variable "我的电脑\\A17031611.lvlib\\设备状态3"(i16 41 ("设备状态")) -> ()  [unwired: 1 in, 1 out]
                  }
                }
                n253 = call "浮动通知.vi"("通知内容"="请安装固定螺栓1并确认扭矩！" ("Status")) -> ()  [unwired: 11 in]
              }
              frame 36 {
                n254 = case shown="2" w855 {
                  tunnel: w854 -> [w857 w870 w874]
                  frame 1 {
                    n255 = Index Array(array=w857, index=1 ("索引")) -> (element=w864:refnum<vi>)
                    n256 = Index Array(array=w857, index=4 ("索引")) -> (element=w858:refnum<vi>)
                    n257 = call "Colour.vi"("result"="OK", "colourRef"=w864) -> ()  [unwired: 9 in, 1 out]
                    n258 = call "Colour.vi"("result"="等待", "colourRef"=w858) -> ()  [unwired: 9 in, 1 out]
                    n259 = call "浮动通知.vi"("通知内容"="请按启动拍照确认电机方向！" ("Status")) -> ()  [unwired: 11 in]
                    n260 = shared-variable "我的电脑\\A17031611.lvlib\\设备状态1"(i16 70 ("设备状态")) -> ()  [unwired: 1 in, 1 out]
                  }
                  frame 2 {
                    n261 = Index Array(array=w870, index #1=0 ("索引")) -> (element #1=w868:refnum<vi>, element #2=w866:refnum<vi>)  [unwired: 2 in, 1 out]
                    n262 = call "Colour -电机.vi"("result"="OK", "colourRef"=w868) -> ()  [unwired: 9 in, 1 out]
                    n263 = call "Colour -电机.vi"("result"="等待", "colourRef"=w866) -> ()  [unwired: 9 in, 1 out]
                    n264 = call "浮动通知.vi"("通知内容"="请安装固定螺栓1并确认扭矩！" ("Status")) -> ()  [unwired: 11 in]
                  }
                  frame Default {
                    n265 = Index Array(array=w874, index #1=1 ("索引")) -> (element #1=w878:refnum<vi>, element #2=w879:refnum<vi>)  [unwired: 1 in]
                    n266 = call "Colour.vi"("result"="OK", "colourRef"=w878) -> ()  [unwired: 9 in, 1 out]
                    n267 = call "浮动通知.vi"("通知内容"="请安装固定螺栓2并确认扭矩！" ("Status")) -> ()  [unwired: 11 in]
                    n268 = call "Colour.vi"("result"="等待", "colourRef"=w879) -> ()  [unwired: 9 in, 1 out]
                    n269 = shared-variable "我的电脑\\A17031611.lvlib\\设备状态3"(i16 40 ("设备状态")) -> ()  [unwired: 1 in, 1 out]
                  }
                }
              }
              frame 40 {
                n270 = control-ref of="电机安装螺栓1扭矩确认"() -> (w880:refnum<vi>)
                n271 = call "Colour -电机.vi"("result"="等待", "colourRef"=w880) -> ()  [unwired: 9 in, 1 out]
                n272 = call "浮动通知.vi"("通知内容"="请安装固定螺栓1并确认扭矩！" ("Status")) -> ()  [unwired: 11 in]
              }
              frame 41 {
                n273 = flat-sequence {
                  frame #0 {
                    n274 = control-ref of="电机安装螺栓1扭矩确认"() -> (w883:refnum<vi>)
                    n275 = call "Colour -电机.vi"("result"="OK", "colourRef"=w883) -> ()  [unwired: 9 in, 1 out]
                  }
                  frame #1 {
                    n276 = local read "电机步骤"() -> (w887:T3)
                    n277 = local write "STEP3"("步骤" ("STEP3")) -> ()
                    n278 = Increment(x=w887) -> (x+1=w888:T3)
                    n279 = Wait (ms)(milliseconds to wait=u32 20 ("等待时间（毫秒）")) -> ()  [unwired: 1 out]
                    n280 = local write "电机步骤"(w888) -> ()
                  }
                }
              }
              frame 42 {
                n281 = control-ref of="电机安装螺栓2扭矩确认"() -> (w890:refnum<vi>)
                n282 = call "浮动通知.vi"("通知内容"="请安装固定螺栓2并确认扭矩！" ("Status")) -> ()  [unwired: 11 in]
                n283 = call "Colour -电机.vi"("result"="等待", "colourRef"=w890) -> ()  [unwired: 9 in, 1 out]
              }
              frame 44 {
                n284 = control-ref of="电机安装螺栓3扭矩确认"() -> (w893:refnum<vi>)
                n285 = call "浮动通知.vi"("通知内容"="请安装固定螺栓3并确认扭矩！" ("Status")) -> ()  [unwired: 11 in]
                n286 = call "Colour -电机.vi"("result"="等待", "colourRef"=w893) -> ()  [unwired: 9 in, 1 out]
              }
              frame 45 {
                n287 = flat-sequence {
                  frame #0 {
                    n288 = control-ref of="电机安装螺栓3扭矩确认"() -> (w895:refnum<vi>)
                    n289 = call "Colour -电机.vi"("result"="OK", "colourRef"=w895) -> ()  [unwired: 9 in, 1 out]
                  }
                  frame #1 {
                    n290 = local read "电机步骤"() -> (w898:T3)
                    n291 = Increment(x=w898) -> (x+1=w899:T3)
                    n292 = local write "STEP3"("步骤" ("STEP3")) -> ()
                    n293 = local write "电机步骤"(w899) -> ()
                    n294 = Wait (ms)(milliseconds to wait=u32 20 ("等待时间（毫秒）")) -> ()  [unwired: 1 out]
                  }
                }
              }
              frame 43 {
                n295 = flat-sequence {
                  frame #0 {
                    n296 = control-ref of="电机安装螺栓2扭矩确认"() -> (w901:refnum<vi>)
                    n297 = call "Colour -电机.vi"("result"="OK", "colourRef"=w901) -> ()  [unwired: 9 in, 1 out]
                  }
                  frame #1 {
                    n298 = local read "电机步骤"() -> (w904:T3)
                    n299 = Increment(x=w904) -> (x+1=w905:T3)
                    n300 = local write "STEP3"("步骤" ("STEP3")) -> ()
                    n301 = local write "电机步骤"(w905) -> ()
                    n302 = Wait (ms)(milliseconds to wait=u32 20 ("等待时间（毫秒）")) -> ()  [unwired: 1 out]
                  }
                }
              }
              frame 51 {
                n303 = case shown="2" w908 {
                  tunnel: w907 -> [_ _ w913]
                  frame 0, 1 {
                  }
                  frame 2 {
                    n304 = call "浮动通知.vi"("通知内容"="请按启动按钮拍照确认！" ("Status")) -> ()  [unwired: 11 in]
                    n305 = shared-variable "我的电脑\\A17031611.lvlib\\设备状态3"(i16 70 ("设备状态")) -> ()  [unwired: 1 in, 1 out]
                  }
                  frame Default {
                    n306 = Index Array(array=w913, index #1=2 ("索引")) -> (element #1=w917:refnum<vi>, element #2=w914:refnum<vi>)  [unwired: 1 in]
                    n307 = call "浮动通知.vi"("通知内容"="请按启动按钮拍照确认！" ("Status")) -> ()  [unwired: 11 in]
                    n308 = call "Colour.vi"("result"="OK", "colourRef"=w917) -> ()  [unwired: 9 in, 1 out]
                    n309 = call "Colour.vi"("result"="等待", "colourRef"=w914) -> ()  [unwired: 9 in, 1 out]
                    n310 = shared-variable "我的电脑\\A17031611.lvlib\\设备状态3"(i16 70 ("设备状态")) -> ()  [unwired: 1 in, 1 out]
                  }
                }
              }
              frame 61 {
                n311 = case shown="默认" w920 {
                  tunnel: w919 -> [w925 _]
                  frame Default {
                    n312 = Index Array(array=w925, index #1=3 ("索引")) -> (element #1=w927:refnum<vi>, element #2=w928:refnum<vi>)  [unwired: 1 in]
                    n313 = call "Colour.vi"("result"="OK", "colourRef"=w927) -> ()  [unwired: 9 in, 1 out]
                    n314 = call "Colour.vi"("result"="等待", "colourRef"=w928) -> ()  [unwired: 9 in, 1 out]
                    n315 = call "浮动通知.vi"("通知内容"="请按启动拍照确认！" ("Status")) -> ()  [unwired: 11 in]
                    n316 = shared-variable "我的电脑\\A17031611.lvlib\\设备状态3"(i16 70 ("设备状态")) -> ()  [unwired: 1 in, 1 out]
                  }
                  frame 0..2 {
                  }
                }
              }
              frame 70 {
                n317 = Index Array(array=w934, index #1=2 ("索引")) -> ()  [unwired: 1 in, 2 out]
                n318 = control-ref of="按启动按钮拍照确认"() -> (w930:refnum<vi>)
                n319 = control-ref of="电机安装螺栓3扭矩确认"() -> (w929:refnum<vi>)
                n320 = call "Colour -电机.vi"("result"="等待", "colourRef"=w930) -> ()  [unwired: 9 in, 1 out]
                n321 = call "Colour -电机.vi"("result"="OK", "colourRef"=w929) -> ()  [unwired: 9 in, 1 out]
              }
              frame 81 {
                n322 = flat-sequence {
                  frame #0 {
                    n323 = control-ref of="按启动按钮拍照确认"() -> (w936:refnum<vi>)
                    n324 = call "Colour -电机.vi"("result"="OK", "colourRef"=w936) -> ()  [unwired: 9 in, 1 out]
                  }
                  frame #1 {
                    n325 = local read "电机步骤"() -> (w939:T3)
                    n326 = Increment(x=w939) -> (x+1=w940:T3)
                    n327 = Wait (ms)(milliseconds to wait=u32 20 ("等待时间（毫秒）")) -> ()  [unwired: 1 out]
                    n328 = local write "STEP3"("步骤" ("STEP3")) -> ()
                    n329 = local write "电机步骤"(w940) -> ()
                  }
                }
              }
              frame 80 {
                n330 = control-ref of="按启动按钮拍照确认"() -> (w942:refnum<vi>)
                n331 = call "Colour -电机.vi"("result"="NG", "colourRef"=w942) -> ()  [unwired: 9 in, 1 out]
                n332 = shared-variable "我的电脑\\A17031611.lvlib\\设备状态3"(i16 70 ("设备状态")) -> ()  [unwired: 1 in, 1 out]
              }
              frame 90 {
                n333 = Index Array(array=w947, index #1=3 ("索引")) -> ()  [unwired: 1 in, 2 out]
                n334 = control-ref of="涂色标"() -> (w945:refnum<vi>)
                n335 = call "浮动通知.vi"("通知内容"="请给固定螺栓涂色标！" ("Status")) -> ()  [unwired: 11 in]
                n336 = call "Colour -电机.vi"("result"="等待", "colourRef"=w945) -> ()  [unwired: 9 in, 1 out]
              }
              frame 91 {
                n337 = flat-sequence {
                  frame #0 {
                    n338 = control-ref of="涂色标"() -> (w949:refnum<vi>)
                    n339 = call "Colour -电机.vi"("result"="OK", "colourRef"=w949) -> ()  [unwired: 9 in, 1 out]
                  }
                  frame #1 {
                    n340 = local read "电机步骤"() -> (w953:T3)
                    n341 = Increment(x=w953) -> (x+1=w954:T3)
                    n342 = local write "STEP3"("步骤" ("STEP3")) -> ()
                    n343 = Wait (ms)(milliseconds to wait=u32 20 ("等待时间（毫秒）")) -> ()  [unwired: 1 out]
                    n344 = local write "电机步骤"(w954) -> ()
                  }
                }
              }
              frame 100 {
                n345 = Index Array(array=w957, index #1=4 ("索引")) -> ()  [unwired: 1 in, 2 out]
                n346 = control-ref of="安装扎带并取走工件"() -> (w956:refnum<vi>)
                n347 = call "Colour -电机.vi"("result"="等待", "colourRef"=w956) -> ()  [unwired: 9 in, 1 out]
                n348 = call "浮动通知.vi"("通知内容"="请安装轧带并取走工件" ("Status")) -> ()  [unwired: 11 in]
              }
              frame 101 {
                n349 = Index Array(array=w960, index #1=5 ("索引")) -> ()  [unwired: 1 in, 2 out]
                n350 = flat-sequence {
                  frame #0 {
                    n351 = control-ref of="安装扎带并取走工件"() -> (w963:refnum<vi>)
                    n352 = call "浮动通知.vi"("通知内容"="完成！" ("Status")) -> ()  [unwired: 11 in]
                    n353 = call "Colour -电机.vi"("result"="OK", "colourRef"=w963) -> ()  [unwired: 9 in, 1 out]
                  }
                  frame #1 {
                    n354 = local read "电机步骤"() -> (w967:T3)
                    n355 = Increment(x=w967) -> (x+1=w966:T3)
                    n356 = local write "STEP3"("步骤" ("STEP3")) -> ()
                    n357 = Wait (ms)(milliseconds to wait=u32 20 ("等待时间（毫秒）")) -> ()  [unwired: 1 out]
                    n358 = local write "电机步骤"(w966) -> ()
                  }
                }
              }
              frame 200 {
                n359 = global read "Global1.vi" "联机模式"() -> (w969:enum16{"单机", "联网"})
                n360 = Wait (ms)(milliseconds to wait=u32 500 ("等待时间（毫秒）")) -> ()  [unwired: 1 out]
                n361 = case shown="\"联网\"" w969 {
                  frame "单机", Default {
                    n362 = global read "Global.vi" "检测结果"() -> (w979:refnum<vi>)
                    n363 = call "浮动通知.vi"("通知内容"="产品合格！" ("Status")) -> ()  [unwired: 11 in]
                    n364 = call "Colour.vi"("result"="OK", "colourRef"=w979) -> ()  [unwired: 9 in, 1 out]
                    n365 = global read "Global.vi" "电机结果显示"() -> (w976:refnum<vi>)
                    n366 = local write "电机步骤"(T3."安装弹簧" ("电机步骤")) -> ()
                    n367 = property class="Str"(reference=w976, "Value"="OK" ("结果显示")) -> (reference out=w975:refnum<vi>)  [unwired: 1 in, 1 out]
                    n368 = shared-variable "我的电脑\\A17031611.lvlib\\设备状态3"(i16 6 ("设备状态")) -> ()  [unwired: 1 in, 1 out]
                    n369 = property class="Str"(reference=w975, "Text.TextColor"=u32 9567230) -> ()  [unwired: 1 in, 2 out]
                  }
                  frame "联网" {
                    n370 = global read "Global.vi" "检测结果"() -> (w981:refnum<vi>)
                    n371 = global write "Global1.vi" "电机工位生产结果"("OK" ("电机工位生产结果")) -> ()
                    n372 = call "浮动通知.vi"("通知内容"="产品合格！" ("Status")) -> ()  [unwired: 11 in]
                    n373 = call "Colour -电机.vi"("result"="OK", "colourRef"=w981) -> ()  [unwired: 9 in, 1 out]
                    n374 = global read "Global.vi" "电机结果显示"() -> (w989:refnum<vi>)
                    n375 = property class="Str"(reference=w989, "Value"="OK" ("结果显示")) -> (reference out=w986:refnum<vi>)  [unwired: 1 in, 1 out]
                    n376 = global read "Global1.vi" "联机模式"() -> (w982:enum16{"单机", "联网"})
                    n377 = property class="Str"(reference=w986, "Text.TextColor"=u32 9567230) -> ()  [unwired: 1 in, 2 out]
                    n378 = case shown="\"联网\"" w982 {
                      tunnel: ["自动" "录入数据库" ("STEP3")] -> w983
                      frame "单机", Default {
                        n379 = shared-variable "我的电脑\\A17031611.lvlib\\设备状态3"(i16 6 ("设备状态")) -> ()  [unwired: 1 in, 1 out]
                        n380 = local write "电机步骤"(T3."安装弹簧" ("电机步骤")) -> ()
                      }
                      frame "联网" {
                      }
                    }
                    n381 = local write "STEP3"(w983) -> ()
                  }
                }
              }
              frame 201 {
                n382 = global read "Global.vi" "检测结果"() -> (w999:refnum<vi>)
                n383 = call "Colour.vi"("result"="NG", "colourRef"=w999) -> ()  [unwired: 9 in, 1 out]
                n384 = call "浮动通知.vi"("通知内容"="产品不合格！" ("Status")) -> ()  [unwired: 11 in]
                n385 = global read "Global.vi" "电机结果显示"() -> (w998:refnum<vi>)
                n386 = property class="Str"(reference=w998, "Value"="NG" ("结果显示")) -> (reference out=w997:refnum<vi>)  [unwired: 1 in, 1 out]
                n387 = property class="Str"(reference=w997, "Text.TextColor"=u32 16711680) -> ()  [unwired: 1 in, 2 out]
              }
              frame 999 {
                n388 = Index Array(array=w1003, index #1=0 ("索引")) -> (element #1=w1011:refnum<vi>, element #2=w1012:refnum<vi>, element #3=w1004:refnum<vi>, element #4=w1001:refnum<vi>)  [unwired: 3 in]
                n389 = call "Colour.vi"("result"="", "colourRef"=w1004) -> ()  [unwired: 9 in, 1 out]
                n390 = call "Colour.vi"("result"="", "colourRef"=w1001) -> ()  [unwired: 9 in, 1 out]
                n391 = call "Colour.vi"("result"="NG", "colourRef"=w1012) -> ()  [unwired: 9 in, 1 out]
                n392 = call "Colour.vi"("result"="OK", "colourRef"=w1011) -> ()  [unwired: 9 in, 1 out]
                n393 = call "浮动通知.vi"("通知内容"="请重新安装固定螺栓！" ("Status")) -> ()  [unwired: 11 in]
                n394 = shared-variable "我的电脑\\A17031611.lvlib\\设备状态3"(i16 40 ("设备状态")) -> ()  [unwired: 1 in, 1 out]
              }
              frame 1024 {
                n395 = call "浮动通知.vi"("通知内容"="急停！" ("Status")) -> ()  [unwired: 11 in]
                n396 = global read "Global.vi" "电机程序自动"() -> (w1014:refnum<vi>)
                n397 = property class="Bool"(reference=w1014, "Value"=FALSE) -> ()  [unwired: 1 in, 2 out]
              }
              frame 3721 {
                n398 = local write "STEP3"("不合格锁定" ("STEP")) -> ()
                n399 = call "浮动通知.vi"("通知内容"="产品不合格程序锁定！" ("Status")) -> ()  [unwired: 11 in]
              }
              frame 3722 {
                n400 = global read "Global.vi" "电机程序自动"() -> (w1019:refnum<vi>)
                n401 = call "浮动通知.vi"("通知内容"="授权成功，请复位！" ("Status")) -> ()  [unwired: 11 in]
                n402 = property class="Bool"(reference=w1019, "Value"=FALSE) -> ()  [unwired: 1 in, 2 out]
              }
              frame 3723 {
                n403 = call "浮动通知.vi"("通知内容"="请取出不合格产品并摆放至不合格品区！" ("Status")) -> ()  [unwired: 11 in]
              }
              frame Default {
              }
            }
          }
          frame "录入数据库" {
            n404 = stacked-sequence {
              frame #0 {
                n405 = Get Date/Time String(date format (0)=enum16{"short", "long", "abbreviated"}."short" ("日期格式(0)"), want seconds? (F)=FALSE ("需要秒？(F)")) -> (date string=w1031:string, time string=w1032:string)  [unwired: 1 in]
                n406 = global read "Global1.vi" "电机工位生产结果"() -> (w1026:string)
                n407 = global read "Global1.vi" "DEVICE_ID"() -> (w1035:string)
                n408 = global read "Global1.vi" "USER_ID"() -> (w1033:string)
                n409 = global read "Global1.vi" "CODE_ID"() -> (w1034:string)
                n410 = Concatenate Strings(w1031, " " ("字符串"), w1032) -> (w1027:string)
                n411 = Decimal String To Number(string=w1035, default (0L)=i64 0 ("默认(0 I32)")) -> (number=w1024:i64)  [unwired: 1 in, 1 out]
                n412 = Decimal String To Number(string=w1033, default (0L)=i64 0 ("默认(0 I32)")) -> (number=w1023:i64)  [unwired: 1 in, 1 out]
                n413 = Decimal String To Number(string=w1034, default (0L)=i64 0 ("默认(0 I32)")) -> (number=w1022:i64)  [unwired: 1 in, 1 out]
                n414 = global read "Global1.vi" "联机模式"() -> (w1042:enum16{"单机", "联网"})
                n415 = Search and Replace String(replace all?=TRUE ("替换全部？(F)"), input string=w1027, search string="/" ("替换字符串(\"\")"), replace string="-" ("替换字符串(\"\")")) -> (result string=w1025:string)  [unwired: 4 in, 3 out]
                n416 = Bundle(w1024, w1023, w1022, "电机工位生产结果"=w1026, "result string"=w1025) -> (w1048:T4)  [unwired: 1 in]
                n417 = call "GetSQLstring.vi"("联机模式"=w1042) -> ("错误输出"=w1045:errorcluster, "连接字符串"=w1044:string)  [unwired: 9 in]
                n418 = Build Array(w1048) -> (w1049:T5)
                n419 = call-poly <vilib>:"DB Tools Open Connection.vi"("error in (no error)"=w1045, "connection information"=w1044) -> ("error out"=w1043:errorcluster, "connection reference"=w1046:T6)  [unwired: 6 in]
                n420 = for {
                  tunnel: w1049 -> [w1054] mode=indexing
                  tunnel: w1046 -> [w1052]
                  shift-right: [w1050] -> w1047
                  shift-left: w1043 -> [w1057]
                  w1053 = string[] ["DEVICE_ID", "USER_ID", "CODE_ID", "RESULT_VALUE", "RESULT_TIME"] ("columns")
                  w1055 = "Result" ("table")
                  n421 = call <vilib>:"DB Tools Insert Data.vi"("data"=w1054, "error in (no error)"=w1057, "columns"=w1053, "table"=w1055, "connection reference"=w1052) -> ("error out"=w1056:errorcluster, "connection reference out"=w1051:T6)  [unwired: 5 in]
                  n422 = case shown="错误" w1056 {
                    selector: w1056 -> [w1058 w1079]
                    tunnel: w1053 -> [_ w1076]
                    tunnel: w1051 -> [w1059 w1068]
                    tunnel: w1055 -> [_ w1080]
                    tunnel: w1054 -> [_ w1072]
                    tunnel: [w1059 w1067] -> _
                    tunnel: [w1058 w1066] -> w1050
                    frame No Error {
                    }
                    frame Error {
                      n423 = Array Subset(array=w1076, index=3 ("长度"), length=2 ("长度")) -> (w1077:string[])
                      n424 = Unbundle(w1072) -> (w1061:i64, w1064:i64, "电机工位生产结果"=w1071:string, "result string"=w1070:string)  [unwired: 1 out]
                      n425 = Number To Decimal String(number=w1064) -> (decimal integer string=w1065:string)  [unwired: 1 in]
                      n426 = Number To Decimal String(number=w1061) -> (decimal integer string=w1060:string)  [unwired: 1 in]
                      n427 = Concatenate Strings("WHERE CODE_ID =" ("condition"), w1065, "AND DEVICE_ID = ", w1060) -> (w1073:string)
                      n428 = Bundle("电机工位生产结果"=w1071, "result string"=w1070) -> (w1069:T7)  [unwired: 1 in]
                      n429 = call <vilib>:"Clear Errors.vi"("error in (no error)"=w1079) -> ("error out"=w1078:errorcluster)  [unwired: 5 in, 1 out]
                      n430 = call <vilib>:"DB Tools Update Data.vi"("condition"=w1073, "data"=w1069, "error in (no error)"=w1078, "columns"=w1077, "table"=w1080, "connection reference"=w1068) -> ("error out"=w1066:errorcluster, "connection reference out"=w1067:T6)  [unwired: 4 in]
                    }
                  }
                }
                n431 = call <vilib>:"Simple Error Handler.vi"("error in (no error)"=w1047) -> ()  [unwired: 4 in, 5 out]
              }
              frame #1 {
                n432 = shared-variable "我的电脑\\Global.lvlib\\工位追溯码"() -> ()  [unwired: 1 in, 2 out]
                n433 = global read "Global1.vi" "电机码"() -> (w1081:string)
                n434 = global read "Global1.vi" "CODE_ID"() -> (w1082:string)
                n435 = Format Into String(format string="UPDATE\ndbo.[Code]\nSET dbo.[Code].CODE_MOTOR = '%s'\n\nWHERE\ndbo.[Code].CODE_ID = %s\n" ("格式字符串"), w1081, w1082) -> (resulting string=w1085:string)  [unwired: 2 in, 1 out]
                n436 = call "SQL_query.vi"("SQL query"=w1085, "联机模式"=enum16{"单机", "联网"}."联网") -> ()  [unwired: 1 in, 3 out]
              }
              frame #2 {
                n437 = call "浮动通知.vi"("通知内容"="电机工位数据录入成功！" ("Status")) -> ()  [unwired: 11 in]
                n438 = local write "电机步骤"(T3."安装弹簧" ("电机步骤")) -> ()
                n439 = shared-variable "我的电脑\\A17031611.lvlib\\设备状态3"(i16 6 ("设备状态")) -> ()  [unwired: 1 in, 1 out]
                n440 = local write "STEP3"("初始化" ("STEP")) -> ()
                n441 = Wait (ms)(milliseconds to wait=u32 500 ("等待时间（毫秒）")) -> ()  [unwired: 1 out]
              }
            }
          }
          frame "不合格锁定" {
            n442 = call "临时授权.vi"() -> ("授权成功"=w1092:bool)  [unwired: 11 in]
            n443 = case shown="真" w1092 {
              frame False {
              }
              frame True {
                n444 = local write "STEP3"("报表" ("STEP")) -> ()
                n445 = shared-variable "我的电脑\\A17031611.lvlib\\设备状态1"(i16 3722 ("设备状态")) -> ()  [unwired: 1 in, 1 out]
              }
            }
            n446 = Wait (ms)(milliseconds to wait=u32 100 ("等待时间（毫秒）")) -> ()  [unwired: 1 out]
          }
          frame "报表" {
            n447 = call "浮动通知.vi"("通知内容"="报表生成中" ("Status")) -> ()  [unwired: 11 in]
            n448 = shared-variable "我的电脑\\Global.lvlib\\工位追溯码"() -> (w1104:string)  [unwired: 1 in, 1 out]
            n449 = Index Array(array="判定结果", index (col)=1 ("禁用的索引 (列)")) -> (element=w1099:bool[])  [unwired: 1 in]
            n450 = And Array Elements(Boolean array=w1099) -> (logical AND=w1096:bool)
            n451 = shared-variable "我的电脑\\Global.lvlib\\联机模式"() -> (w1101:i16)  [unwired: 1 in, 1 out]
            n452 = call "Report_A170316-11.vi"("文件重命名"=TRUE, "文件名称"=w1104, "布尔数组"="判定结果") -> ("error out"=w1102:errorcluster)  [unwired: 8 in]
            n453 = case shown="真" w1096 {
              frame False {
              }
              frame True {
                n454 = global read "Global.vi" "电机生产数量"() -> (w1113:refnum<vi>)
                n455 = property class="Num"(reference=w1113) -> (reference out=w1112:refnum<vi>, error out=w1111:errorcluster, "Value"=w1110:variant)  [unwired: 1 in]
                n456 = Variant To Data(type=u32 0, Variant=w1110) -> (data=w1109:u32)  [unwired: 1 in, 1 out]
                n457 = Increment(x=w1109) -> (x+1=w1108:u32)
                n458 = property class="Num"(reference=w1112, error in=w1111, "Value"=w1108) -> ()  [unwired: 2 out]
              }
            }
            n459 = case shown="0, 默认" w1101 {
              tunnel: w1102 -> [_ w1114]
              frame 0, Default {
              }
              frame 1 {
                n460 = call "上传数据库.vi"("错误输入"=w1114) -> ()  [unwired: 10 in, 1 out]
              }
            }
            n461 = shared-variable "我的电脑\\A17031611.lvlib\\设备状态1"() -> (w1095:i16)  [unwired: 1 in, 1 out]
            n462 = case shown="3721..3723" w1095 {
              frame Default {
                n463 = local write "STEP3"("初始化" ("STEP")) -> ()
              }
              frame 3721..3723 {
                n464 = local write "STEP3"("等待" ("STEP")) -> ()
              }
            }
          }
          frame "步骤" {
            n465 = case shown="\"安装弹簧\", 默认" "电机步骤" {
              selector: "电机步骤" -> [w1118 _]
              tunnel: [w1117 "等待"] -> w1115
              frame "安装弹簧", Default {
                n466 = global read "Global.vi" "电机安装"() -> (w1120:bool[])
                n467 = Index Array(array=w1120, index=w1118) -> (element=w1119:bool)
                n468 = case shown="真" w1119 {
                  tunnel: w1118 -> [_ w1125]
                  tunnel: ["步骤" w1124] -> w1117
                  frame False {
                    n469 = local read "电机步骤"() -> (w1123:T3)
                    n470 = Increment(x=w1123) -> (x+1=w1122:T3)
                    n471 = local write "电机步骤"(w1122) -> ()
                  }
                  frame True {
                    n472 = case shown="\"电机螺栓2\"" w1125 {
                      tunnel: ["等待" "等待" "等待" "扫电机码" "等待" "等待" "等待" "等待" "等待" "等待"] -> w1124
                      frame "安装弹簧", Default {
                        n473 = shared-variable "我的电脑\\A17031611.lvlib\\设备状态3"(i16 16 ("设备状态")) -> ()  [unwired: 1 in, 1 out]
                      }
                      frame "安装O型圈" {
                        n474 = shared-variable "我的电脑\\A17031611.lvlib\\设备状态3"(i16 18 ("设备状态")) -> ()  [unwired: 1 in, 1 out]
                      }
                      frame "安装弹性垫圈" {
                        n475 = shared-variable "我的电脑\\A17031611.lvlib\\设备状态3"(i16 20 ("设备状态")) -> ()  [unwired: 1 in, 1 out]
                      }
                      frame "电机螺栓1" {
                      }
                      frame "电机螺栓2" {
                        n476 = shared-variable "我的电脑\\A17031611.lvlib\\设备状态3"(i16 42 ("设备状态控制字")) -> ()  [unwired: 1 in, 1 out]
                      }
                      frame "电机螺栓3" {
                        n477 = shared-variable "我的电脑\\A17031611.lvlib\\设备状态3"(i16 44 ("设备状态控制字")) -> ()  [unwired: 1 in, 1 out]
                      }
                      frame "电机拍照" {
                        n478 = shared-variable "我的电脑\\A17031611.lvlib\\设备状态3"(i16 70 ("设备状态控制字")) -> ()  [unwired: 1 in, 1 out]
                      }
                      frame "涂色标" {
                        n479 = shared-variable "我的电脑\\A17031611.lvlib\\设备状态3"(i16 90 ("设备状态控制字")) -> ()  [unwired: 1 in, 1 out]
                      }
                      frame "装轧带" {
                        n480 = shared-variable "我的电脑\\A17031611.lvlib\\设备状态3"(i16 90 ("设备状态控制字")) -> ()  [unwired: 1 in, 1 out]
                      }
                      frame "取走工件" {
                        n481 = shared-variable "我的电脑\\A17031611.lvlib\\设备状态3"(i16 100 ("设备状态控制字")) -> ()  [unwired: 1 in, 1 out]
                      }
                    }
                  }
                }
              }
              frame "完成" {
                n482 = shared-variable "我的电脑\\A17031611.lvlib\\设备状态3"(i16 200 ("设备状态控制字")) -> ()  [unwired: 1 in, 1 out]
              }
            }
            n483 = local write "STEP3"(w1115) -> ()
          }
        }
        n484 = global read "Global.vi" "程序关闭"() -> (w633:bool)
      }
      n485 = while {
        stop <- w53 stop-if-true
        n486 = Wait Until Next ms Multiple(millisecond multiple=u32 10 ("毫秒倍数")) -> ()  [unwired: 1 out]
        n487 = case shown="\"自动\"" "STEP2" {
          frame "等待", Default {
            n488 = local write "STEP2"("自动" ("STEP")) -> ()
          }
          frame "手动" {
          }
          frame "初始化" {
            n489 = stacked-sequence {
              frame #0 {
                w179 = enum16{"录入", "清空"}."清空" ("功能")
                n490 = global read "Global.vi" "安装支架生产数量"() -> (w171:refnum<vi>)
                n491 = shared-variable "我的电脑\\Global.lvlib\\工位追溯码"("" ("传感器码")) -> ()  [unwired: 1 in, 1 out]
                n492 = call "物料信息录入.vi"("功能"=w179) -> ("错误输出"=w178:errorcluster)  [unwired: 14 in]
                n493 = call "质量信息录入.vi"("功能"=w179, "错误输入（无错误）"=w178) -> ("错误输出"=w180:errorcluster)  [unwired: 13 in]
                n494 = property class="Num"(reference=w171, "Value"=0 ("磨合次数")) -> ()  [unwired: 1 in, 2 out]
                n495 = call "不合格信息录入.vi"("功能"=w179, "错误输入（无错误）"=w180) -> ()  [unwired: 13 in, 1 out]
                n496 = global read "Global.vi" "ECU自动"() -> (w176:refnum<vi>)
                n497 = global read "Global.vi" "检测结果"() -> (w174:refnum<vi>)
                n498 = property class="Bool (严格)"(reference=w176, "Value"=TRUE) -> ()  [unwired: 1 in, 2 out]
                n499 = shared-variable "我的电脑\\A17031611.lvlib\\设备状态2"(i16 6 ("设备状态")) -> ()  [unwired: 1 in, 1 out]
                n500 = call "Colour.vi"("result"="", "colourRef"=w174) -> ()  [unwired: 9 in, 1 out]
              }
              frame #1 {
                n501 = local write "ECU步骤"(T2."控制器安装螺栓1" ("ECU步骤")) -> ()
              }
              frame #2 {
                n502 = local write "STEP2"("等待" ("STEP2")) -> ()
              }
            }
          }
          frame "扫主码" {
            n503 = stacked-sequence {
              frame #0 {
                w184 = "请扫ECU工位主码！" ("提示信息")
                n504 = call "浮动通知2.vi"("通知内容"=w184) -> ()  [unwired: 11 in]
                n505 = call "输入框.vi"("提示信息"=w184) -> ("条形码输出"=w185:string)
                n506 = case shown="\"\", 默认" w185 {
                  selector: w185 -> [w186 _]
                  tunnel: [w187 "手动"] -> w183
                  frame "", Default {
                    n507 = shared-variable "我的电脑\\Global.lvlib\\工位追溯码_ECU"(w186) -> ()  [unwired: 1 in, 1 out]
                    n508 = global write "Global1.vi" "工位追溯码_ECU"(w186) -> ()
                    n509 = global read "Global1.vi" "联机模式"() -> (w188:enum16{"单机", "联网"})
                    n510 = case shown="\"联网\"" w188 {
                      tunnel: w186 -> [_ w191]
                      tunnel: ["控制器扫码" ("State(s) in Front (\"\")") w190] -> w187
                      frame "单机", Default {
                      }
                      frame "联网" {
                        n511 = stacked-sequence {
                          tunnel: w191 -> [w192 _ _]
                          tunnel: [_ _ w212] -> w190
                          frame #0 {
                            n512 = global read "Global1.vi" "PRODUCT_ID_ECU"() -> (w196:string)
                            n513 = Format Into String "格式化写入字符串"(format string="SELECT\ndbo.[Code].CODE_ID\nFROM\ndbo.[Code]\nWHERE\ndbo.[Code].CODE_MAIN = '%s'\nAND\ndbo.[Code].PRODUCT_ID = %s\n" ("格式字符串"), w192, w196) -> (resulting string=w198:string)  [unwired: 2 in, 1 out]
                            n514 = call "SQL_query.vi"("SQL query"=w198, "联机模式"=enum16{"单机", "联网"}."联网") -> ("data"=w201:string[][])  [unwired: 1 in, 2 out]
                            n515 = Index Array(array=w201, index (row)=0 ("索引 (行)")) -> (element=w200:string[])  [unwired: 1 in]
                            n516 = Index Array(array=w200, index=0 ("索引")) -> (element=w193:string)
                            n517 = global write "Global1.vi" "CODE_ID_ECU"(w193) -> ()
                          }
                          frame #1 {
                            n518 = global read "Global1.vi" "前序DEVICE_ID_ECU"() -> (w202:string)
                            n519 = global read "Global1.vi" "CODE_ID_ECU"() -> (w203:string)
                            n520 = Format Into String(format string="SELECT\ndbo.[Result].RESULT_VALUE\nFROM\ndbo.[Result]\nWHERE\ndbo.[Result].DEVICE_ID = %s\nAND\ndbo.[Result].CODE_ID = %s\n" ("格式字符串"), w202, w203) -> (resulting string=w205:string)  [unwired: 2 in, 1 out]
                            n521 = call "SQL_query.vi"("SQL query"=w205, "联机模式"=enum16{"单机", "联网"}."联网") -> ("data"=w211:string[][])  [unwired: 1 in, 2 out]
                            n522 = Index Array(array=w211, index (row)=0 ("索引 (行)")) -> (element=w210:string[])  [unwired: 1 in]
                            n523 = Index Array(array=w210, index=0 ("索引")) -> (element=w204:string)
                            n524 = local write "前序OK？_ECU"(w204) -> ()
                          }
                          frame #2 {
                            n525 = local read "前序OK？_ECU"() -> (w213:string)
                            n526 = case shown="\"OK\"" w213 {
                              tunnel: ["控制器扫码" "自动" "自动"] -> w212
                              frame "OK" {
                                n527 = global read "Global.vi" "ECU前序显示字"() -> (w216:refnum<vi>)
                                n528 = global read "Global1.vi" "ECU上序状态"() -> (w215:refnum<vi>)
                                n529 = property class="Str"(reference=w216, "Value"="OK" ("值")) -> ()  [unwired: 1 in, 2 out]
                                n530 = call "Colour -ECU.vi"("result"="OK", "colourRef"=w215) -> ()  [unwired: 9 in, 1 out]
                              }
                              frame Default {
                                n531 = global read "Global1.vi" "ECU上序状态"() -> (w222:refnum<vi>)
                                n532 = Wait (ms)(milliseconds to wait=u32 3000 ("等待时间（毫秒）")) -> ()  [unwired: 1 out]
                                n533 = call "浮动通知2.vi"("通知内容"="ECU工位上序漏序！" ("Status")) -> ()  [unwired: 11 in]
                                n534 = global read "Global.vi" "ECU前序显示字"() -> (w219:refnum<vi>)
                                n535 = call "Colour.vi"("result"="等待", "colourRef"=w222) -> ()  [unwired: 9 in, 1 out]
                                n536 = shared-variable "我的电脑\\A17031611.lvlib\\设备状态2"(i16 6 ("设备状态控制字")) -> ()  [unwired: 1 in, 1 out]
                                n537 = property class="Str"(reference=w219, "Value"="漏序" ("值")) -> ()  [unwired: 1 in, 2 out]
                              }
                              frame "NG" {
                                n538 = Wait (ms)(milliseconds to wait=u32 3000 ("等待时间（毫秒）")) -> ()  [unwired: 1 out]
                                n539 = global read "Global1.vi" "ECU上序状态"() -> (w228:refnum<vi>)
                                n540 = call "浮动通知2.vi"("通知内容"="上序生产结果不合格！" ("Status")) -> ()  [unwired: 11 in]
                                n541 = global read "Global.vi" "ECU前序显示字"() -> (w230:refnum<vi>)
                                n542 = call "Colour -ECU.vi"("result"="NG", "colourRef"=w228) -> ()  [unwired: 9 in, 1 out]
                                n543 = shared-variable "我的电脑\\A17031611.lvlib\\设备状态2"(i16 6 ("设备状态控制字")) -> ()  [unwired: 1 in, 1 out]
                                n544 = property class="Str"(reference=w230, "Value"="NG" ("值")) -> ()  [unwired: 1 in, 2 out]
                              }
                            }
                          }
                        }
                      }
                    }
                  }
                  frame "exit" {
                  }
                }
                n545 = local write "STEP2"(w183) -> ()
              }
              frame #1 {
                n546 = Wait (ms)(milliseconds to wait=u32 100 ("等待时间（毫秒）")) -> ()  [unwired: 1 out]
              }
            }
          }
          frame "控制器扫码" {
            n547 = stacked-sequence {
              frame #0 {
                w237 = "请扫请控制器码！！" ("提示信息")
                n548 = call "输入框.vi"("提示信息"=w237) -> ("条形码输出"=w238:string)
                n549 = call "浮动通知2.vi"("通知内容"=w237) -> ()  [unwired: 11 in]
                n550 = case shown="\"\", 默认" w238 {
                  selector: w238 -> [w244 _]
                  tunnel: [w247 "手动"] -> w239
                  frame "", Default {
                    n551 = global read "Global.vi" "硬件版本号"() -> (w240:string)
                    n552 = global write "Global1.vi" "控制器码"(w244) -> ()
                    n553 = shared-variable "我的电脑\\Global.lvlib\\控制器码"(w244) -> ()  [unwired: 1 in, 1 out]
                    n554 = xnode "匹配正则表达式"("输入字符串"=w244, "正则表达式"="-") -> ("匹配之前"=w242:string)  [unwired: 4 in, 4 out]
                    n555 = call <vilib>:"Trim Whitespace.vi"("string"=w242) -> ("trimmed string"=w245:string)  [unwired: 1 in]
                    n556 = call <vilib>:"Trim Whitespace.vi"("string"=w240) -> ("trimmed string"=w246:string)  [unwired: 1 in]
                    n557 = Equal?(x=w245, y=w246) -> (x = y?=w241:bool)
                    n558 = case shown="真" w241 {
                      tunnel: ["控制器扫码" ("State(s) in Front (\"\")") w367] -> w247
                      frame False {
                        w365 = 0 items=["OK", "OKCancel", "AbortRetryIgnore", "YesNoCancel", "YesNo", "RetryCancel"] ("buttons")
                        w366 = 16 items=["None"=0, "Hand, Error, Stop"=16, "Question"=32, "Exclamation, Warning"=48, "Asterisk, Information"=64] ("icon")
                        n559 = call "信息框（标题、文本、图标）.vi"("icon"=w366, "buttons"=w365, "caption"="控制器混料", "text"="混料请核对控制器!") -> ()  [unwired: 6 in, 2 out]
                      }
                      frame True {
                        n560 = global read "Global1.vi" "联机模式"() -> (w368:enum16{"单机", "联网"})
                        n561 = case shown="\"单机\", 默认" w368 {
                          tunnel: ["步骤" ("State(s) in Front (\"\")") "步骤"] -> w367
                          frame "单机", Default {
                            n562 = global read "Global.vi" "安装支架生产数量"() -> (w372:refnum<vi>)
                            n563 = property class="Num"(reference=w372) -> (reference out=w373:refnum<vi>, error out=w374:errorcluster, "Value"=w375:variant)  [unwired: 1 in]
                            n564 = Variant To Data(type=u32 0, Variant=w375) -> (data=w376:u32)  [unwired: 1 in, 1 out]
                            n565 = Increment(x=w376) -> (x+1=w377:u32)
                            n566 = property class="Num"(reference=w373, error in=w374, "Value"=w377) -> ()  [unwired: 2 out]
                            n567 = Wait (ms)(milliseconds to wait=u32 10 ("等待时间（毫秒）")) -> ()  [unwired: 1 out]
                          }
                          frame "联网" {
                            n568 = global read "Global.vi" "安装支架生产数量"() -> (w379:refnum<vi>)
                            n569 = property class="Num"(reference=w379) -> (reference out=w380:refnum<vi>, error out=w381:errorcluster, "Value"=w382:variant)  [unwired: 1 in]
                            n570 = Variant To Data "变体至数据转换"(type=u32 0, Variant=w382) -> (data=w383:u32)  [unwired: 1 in, 1 out]
                            n571 = Increment(x=w383) -> (x+1=w384:u32)
                            n572 = property class="Num"(reference=w380, error in=w381, "Value"=w384) -> ()  [unwired: 2 out]
                          }
                        }
                      }
                    }
                  }
                  frame "exit" {
                  }
                }
                n573 = local write "STEP2"(w239) -> ()
              }
              frame #1 {
                n574 = Wait (ms)(milliseconds to wait=u32 100 ("等待时间（毫秒）")) -> ()  [unwired: 1 out]
              }
            }
          }
          frame "自动" {
            # "3=41\n2=42\n1=43\n0=45"
            # "4=31\n3=32\n2=33\n1=34\n0=35"
            n575 = shared-variable "我的电脑\\A17031611.lvlib\\安装支架螺栓2"() -> (w388:u16)  [unwired: 1 in, 1 out]
            n576 = shared-variable "我的电脑\\A17031611.lvlib\\安装支架螺栓数"() -> (w389:u16)  [unwired: 1 in, 1 out]
            n577 = shared-variable "我的电脑\\A17031611.lvlib\\设备状态2"() -> (w390:i16)  [unwired: 1 in, 1 out]
            n578 = global read "A170316-11.vi" "安装支架LED"() -> (w391:refnum<vi>[])
            n579 = case shown="6" w390 {
              tunnel: w391 -> [_ _ _ _ _ w395 _ w403 _ _ _ _ _ _ _ _ _ _ _ _ _ _ _ w469 w471 _ _ w487 w490 w497 _ _ w524 _ _ _ _]
              tunnel: w389 -> [_ _ _ _ _ _ _ w404 _ _ _ _ _ _ _ _ _ _ _ _ _ _ _ _ _ _ _ _ _ _ _ _ _ _ _ _ _]
              tunnel: w388 -> [_ _ _ _ _ _ _ _ _ _ _ _ _ _ _ _ _ _ _ _ _ _ _ _ _ _ _ _ _ _ _ _ _ _ _ _ _]
              frame Default {
              }
              frame -128 {
                n580 = global read "Global.vi" "ECU自动"() -> (w393:refnum<vi>)
                n581 = property class="Bool (严格)"(reference=w393, "Value"=FALSE) -> ()  [unwired: 1 in, 2 out]
              }
              frame 5 {
                (unwired) "ECU工位复位完成！" ("Status")
              }
              frame 6 {
                n582 = local write "STEP2"("初始化" ("STEP2")) -> ()
              }
              frame 0 {
                (unwired) "手动状态！" ("Status")
              }
              frame 7 {
                n583 = for {
                  tunnel: w395 -> [w402] mode=indexing
                  n584 = call "Colour -ECU.vi"("result"="", "colourRef"=w402) -> ()  [unwired: 9 in, 1 out]
                }
                n585 = global read "Global.vi" "ECU结果显示"() -> (w397:refnum<vi>)
                n586 = property class="Str"(reference=w397, "Value"="..." ("结果显示")) -> (reference out=w398:refnum<vi>)  [unwired: 1 in, 1 out]
                n587 = property class="Str"(reference=w398, "Text.TextColor"=u32 16776960) -> ()  [unwired: 1 in, 2 out]
                n588 = local write "STEP2"("扫主码" ("STEP2")) -> ()
              }
              frame 9 {
              }
              frame 10 {
                n589 = case shown="2" w404 {
                  tunnel: w403 -> [_ _ _ _ _]
                  frame 0, Default {
                    n590 = shared-variable "我的电脑\\A17031611.lvlib\\设备状态2"(i16 35 ("设备状态")) -> ()  [unwired: 1 in, 1 out]
                  }
                  frame 1 {
                    n591 = shared-variable "我的电脑\\A17031611.lvlib\\设备状态2"(i16 34 ("设备状态")) -> ()  [unwired: 1 in, 1 out]
                  }
                  frame 2 {
                    n592 = shared-variable "我的电脑\\A17031611.lvlib\\设备状态2"(i16 33 ("设备状态")) -> ()  [unwired: 1 in, 1 out]
                  }
                  frame 3 {
                    n593 = shared-variable "我的电脑\\A17031611.lvlib\\设备状态2"(i16 32 ("设备状态")) -> ()  [unwired: 1 in, 1 out]
                  }
                  frame 4 {
                    n594 = shared-variable "我的电脑\\A17031611.lvlib\\设备状态2"(i16 31 ("设备状态")) -> ()  [unwired: 1 in, 1 out]
                  }
                }
              }
              frame 31 {
                n595 = control-ref of="控制器安装螺栓1拧紧确认"() -> (w411:refnum<vi>)
                n596 = call "浮动通知2.vi"("通知内容"="请安装固定螺栓1并确认扭矩！" ("Status")) -> ()  [unwired: 11 in]
                n597 = call "Colour -ECU.vi"("result"="等待", "colourRef"=w411) -> ()  [unwired: 9 in, 1 out]
              }
              frame 32 {
                n598 = flat-sequence {
                  frame #0 {
                    n599 = control-ref of="控制器安装螺栓1拧紧确认"() -> (w413:refnum<vi>)
                    n600 = call "Colour.vi"("result"="OK", "colourRef"=w413) -> ()  [unwired: 9 in, 1 out]
                  }
                  frame #1 {
                    n601 = local read "ECU步骤"() -> (w417:T2)
                    n602 = Increment(x=w417) -> (x+1=w416:T2)
                    n603 = local write "STEP2"("步骤" ("STEP2")) -> ()
                    n604 = local write "ECU步骤"(w416) -> ()
                  }
                }
              }
              frame 33 {
                n605 = control-ref of="控制器安装螺栓2拧紧确认"() -> (w419:refnum<vi>)
                n606 = call "浮动通知2.vi"("通知内容"="控制器安装螺栓2拧紧确认！" ("Status")) -> ()  [unwired: 11 in]
                n607 = call "Colour -ECU.vi"("result"="等待", "colourRef"=w419) -> ()  [unwired: 9 in, 1 out]
              }
              frame 34 {
                n608 = flat-sequence {
                  frame #0 {
                    n609 = control-ref of="控制器安装螺栓2拧紧确认"() -> (w422:refnum<vi>)
                    n610 = call "Colour -ECU.vi"("result"="OK", "colourRef"=w422) -> ()  [unwired: 9 in, 1 out]
                  }
                  frame #1 {
                    n611 = local read "ECU步骤"() -> (w425:T2)
                    n612 = Increment(x=w425) -> (x+1=w424:T2)
                    n613 = local write "STEP2"("步骤" ("STEP2")) -> ()
                    n614 = local write "ECU步骤"(w424) -> ()
                  }
                }
              }
              frame 35 {
                n615 = control-ref of="控制器安装螺栓3拧紧确认"() -> (w427:refnum<vi>)
                n616 = call "浮动通知2.vi"("通知内容"="控制器安装螺栓3拧紧确认!") -> ()  [unwired: 11 in]
                n617 = call "Colour -ECU.vi"("result"="等待", "colourRef"=w427) -> ()  [unwired: 9 in, 1 out]
              }
              frame 36 {
                n618 = flat-sequence {
                  frame #0 {
                    n619 = control-ref of="控制器安装螺栓3拧紧确认"() -> (w430:refnum<vi>)
                    n620 = call "Colour -ECU.vi"("result"="等待", "colourRef"=w430) -> ()  [unwired: 9 in, 1 out]
                  }
                  frame #1 {
                    n621 = local read "ECU步骤"() -> (w433:T2)
                    n622 = local write "STEP2"("步骤" ("STEP2")) -> ()
                    n623 = Increment(x=w433) -> (x+1=w432:T2)
                    n624 = local write "ECU步骤"(w432) -> ()
                  }
                }
              }
              frame 40 {
              }
              frame 41 {
                n625 = control-ref of="安装支架螺栓1拧紧确认"() -> (w435:refnum<vi>)
                n626 = call "浮动通知2.vi"("通知内容"="请安装控制器支架1并确认扭矩！" ("Status")) -> ()  [unwired: 11 in]
                n627 = call "Colour -ECU.vi"("result"="等待", "colourRef"=w435) -> ()  [unwired: 9 in, 1 out]
              }
              frame 42 {
                n628 = flat-sequence {
                  frame #0 {
                    n629 = control-ref of="安装支架螺栓1拧紧确认"() -> (w438:refnum<vi>)
                    n630 = call "Colour -ECU.vi"("result"="OK", "colourRef"=w438) -> ()  [unwired: 9 in, 1 out]
                  }
                  frame #1 {
                    n631 = local read "ECU步骤"() -> (w441:T2)
                    n632 = Increment(x=w441) -> (x+1=w440:T2)
                    n633 = local write "STEP2"("步骤" ("STEP2")) -> ()
                    n634 = local write "ECU步骤"(w440) -> ()
                  }
                }
              }
              frame 43 {
                n635 = control-ref of="安装支架螺栓2拧紧确认"() -> (w443:refnum<vi>)
                n636 = call "Colour -ECU.vi"("result"="等待", "colourRef"=w443) -> ()  [unwired: 9 in, 1 out]
                n637 = call "浮动通知2.vi"("通知内容"="请安装控制器支架2并确认扭矩！" ("Status")) -> ()  [unwired: 11 in]
              }
              frame 44 {
                n638 = flat-sequence {
                  frame #0 {
                    n639 = control-ref of="安装支架螺栓2拧紧确认"() -> (w446:refnum<vi>)
                    n640 = call "Colour -ECU.vi"("result"="OK", "colourRef"=w446) -> ()  [unwired: 9 in, 1 out]
                  }
                  frame #1 {
                    n641 = local read "ECU步骤"() -> (w448:T2)
                    n642 = Increment(x=w448) -> (x+1=w449:T2)
                    n643 = local write "STEP2"("步骤" ("STEP2")) -> ()
                    n644 = local write "ECU步骤"(w449) -> ()
                  }
                }
              }
              frame 45 {
                n645 = control-ref of="安装支架螺栓3拧紧确认"() -> (w451:refnum<vi>)
                n646 = call "浮动通知2.vi"("通知内容"="请安装控制器支架3并确认扭矩") -> ()  [unwired: 11 in]
                n647 = call "Colour -ECU.vi"("result"="等待", "colourRef"=w451) -> ()  [unwired: 9 in, 1 out]
              }
              frame 46 {
                n648 = flat-sequence {
                  frame #0 {
                    n649 = control-ref of="安装支架螺栓3拧紧确认"() -> (w454:refnum<vi>)
                    n650 = call "Colour -ECU.vi"("result"="OK", "colourRef"=w454) -> ()  [unwired: 9 in, 1 out]
                  }
                  frame #1 {
                    n651 = local read "ECU步骤"() -> (w456:T2)
                    n652 = Increment(x=w456) -> (x+1=w457:T2)
                    n653 = local write "STEP2"("步骤" ("STEP2")) -> ()
                    n654 = local write "ECU步骤"(w457) -> ()
                  }
                }
              }
              frame 47 {
                n655 = control-ref of="安装支架螺栓4拧紧确认"() -> (w459:refnum<vi>)
                n656 = call "浮动通知2.vi"("通知内容"="请安装控制器支架3并确认扭矩") -> ()  [unwired: 11 in]
                n657 = call "Colour -ECU.vi"("result"="等待", "colourRef"=w459) -> ()  [unwired: 9 in, 1 out]
              }
              frame 48 {
                n658 = flat-sequence {
                  frame #0 {
                    n659 = control-ref of="安装支架螺栓4拧紧确认"() -> (w462:refnum<vi>)
                    n660 = call "Colour -ECU.vi"("result"="OK", "colourRef"=w462) -> ()  [unwired: 9 in, 1 out]
                  }
                  frame #1 {
                    n661 = local read "ECU步骤"() -> (w464:T2)
                    n662 = Increment(x=w464) -> (x+1=w465:T2)
                    n663 = local write "STEP2"("步骤" ("STEP2")) -> ()
                    n664 = local write "ECU步骤"(w465) -> ()
                  }
                }
              }
              frame 60 {
                n665 = Index Array(array=w469, index=4 ("索引")) -> ()  [unwired: 1 out]
                n666 = call "浮动通知2.vi"("通知内容"="请取记号笔标记!") -> ()  [unwired: 11 in]
                n667 = control-ref of="安装支架涂色标"() -> (w467:refnum<vi>)
                n668 = call "Colour -ECU.vi"("result"="等待", "colourRef"=w467) -> ()  [unwired: 9 in, 1 out]
              }
              frame 61 {
                n669 = Index Array(array=w471, index #1=4 ("索引")) -> ()  [unwired: 1 in, 2 out]
                n670 = flat-sequence {
                  frame #0 {
                    n671 = control-ref of="安装支架涂色标"() -> (w473:refnum<vi>)
                    n672 = call "Colour.vi"("result"="OK", "colourRef"=w473) -> ()  [unwired: 9 in, 1 out]
                  }
                  frame #1 {
                    n673 = local read "ECU步骤"() -> (w476:T2)
                    n674 = Increment(x=w476) -> (x+1=w477:T2)
                    n675 = local write "STEP2"("步骤" ("STEP2")) -> ()
                    n676 = local write "ECU步骤"(w477) -> ()
                  }
                }
              }
              frame 70 {
                n677 = control-ref of="安装支架线卡扎带安装"() -> (w479:refnum<vi>)
                n678 = call "Colour -ECU.vi"("result"="等待", "colourRef"=w479) -> ()  [unwired: 9 in, 1 out]
                n679 = call "浮动通知2.vi"("通知内容"="请取轧带！" ("Status")) -> ()  [unwired: 11 in]
              }
              frame 71 {
                n680 = flat-sequence {
                  frame #0 {
                    n681 = control-ref of="安装支架线卡扎带安装"() -> (w483:refnum<vi>)
                    n682 = call "浮动通知2.vi"("通知内容"="完成！" ("Status")) -> ()  [unwired: 11 in]
                    n683 = call "Colour -ECU.vi"("result"="OK", "colourRef"=w483) -> ()  [unwired: 9 in, 1 out]
                  }
                  frame #1 {
                    n684 = local write "STEP2"("步骤" ("STEP2")) -> ()
                    n685 = local write "ECU步骤"(T2."完成" ("ECU步骤")) -> ()
                  }
                }
              }
              frame 81 {
                n686 = Index Array(array=w487, index #1=8 ("索引")) -> ()  [unwired: 1 in, 2 out]
                n687 = call "浮动通知2.vi"("通知内容"="完成!") -> ()  [unwired: 11 in]
                n688 = shared-variable "我的电脑\\A17031611.lvlib\\设备状态2"(i16 200 ("设备状态")) -> ()  [unwired: 1 in, 1 out]
              }
              frame 91 {
                (unwired) "请安装电机扎带并取走工件！" ("Status")
                n689 = Index Array(array=w490, index #1=5 ("索引")) -> (element #1=w492:refnum<vi>, element #2=w491:refnum<vi>)  [unwired: 1 in]
                n690 = call "Colour.vi"("result"="OK", "colourRef"=w492) -> ()  [unwired: 9 in, 1 out]
                n691 = call "Colour.vi"("result"="等待", "colourRef"=w491) -> ()  [unwired: 9 in, 1 out]
                n692 = shared-variable "我的电脑\\A17031611.lvlib\\设备状态3"(i16 100 ("设备状态")) -> ()  [unwired: 1 in, 1 out]
              }
              frame 101 {
                (unwired) "完成！" ("Status")
                n693 = Index Array(array=w497, index #1=6 ("索引")) -> (element #1=w499:refnum<vi>, element #2=w498:refnum<vi>)  [unwired: 1 in]
                n694 = call "Colour.vi"("result"="OK", "colourRef"=w499) -> ()  [unwired: 9 in, 1 out]
                n695 = call "Colour.vi"("result"="等待", "colourRef"=w498) -> ()  [unwired: 9 in, 1 out]
                n696 = shared-variable "我的电脑\\A17031611.lvlib\\设备状态3"(i16 110 ("设备状态")) -> ()  [unwired: 1 in, 1 out]
              }
              frame 200 {
                n697 = global read "Global.vi" "检测结果"() -> (w513:refnum<vi>)
                n698 = global write "Global1.vi" "ECU工位生产结果"("OK" ("电机工位生产结果")) -> ()
                n699 = call "浮动通知2.vi"("通知内容"="产品合格！" ("Status")) -> ()  [unwired: 11 in]
                n700 = call "Colour.vi"("result"="OK", "colourRef"=w513) -> ()  [unwired: 9 in, 1 out]
                n701 = global read "Global.vi" "ECU结果显示"() -> (w511:refnum<vi>)
                n702 = property class="Str"(reference=w511, "Value"="OK" ("结果显示")) -> (reference out=w508:refnum<vi>)  [unwired: 1 in, 1 out]
                n703 = global read "Global1.vi" "联机模式"() -> (w505:enum16{"单机", "联网"})
                n704 = property class="Str"(reference=w508, "Text.TextColor"=u32 9567230) -> ()  [unwired: 1 in, 2 out]
                n705 = case shown="\"联网\"" w505 {
                  tunnel: ["自动" "录入数据库" ("STEP3")] -> w504
                  frame "单机", Default {
                    n706 = shared-variable "我的电脑\\A17031611.lvlib\\设备状态2"(i16 6 ("设备状态")) -> ()  [unwired: 1 in, 1 out]
                    n707 = local write "ECU步骤"(T2."控制器安装螺栓1" ("ECU步骤")) -> ()
                  }
                  frame "联网" {
                  }
                }
                n708 = local write "STEP2"(w504) -> ()
              }
              frame 201 {
                (unwired) "产品不合格！" ("Status")
                n709 = global read "Global.vi" "检测结果"() -> (w522:refnum<vi>)
                n710 = call "Colour.vi"("result"="NG", "colourRef"=w522) -> ()  [unwired: 9 in, 1 out]
                n711 = global read "Global.vi" "电机结果显示"() -> (w521:refnum<vi>)
                n712 = property class="Str"(reference=w521, "Value"="NG" ("结果显示")) -> (reference out=w520:refnum<vi>)  [unwired: 1 in, 1 out]
                n713 = property class="Str"(reference=w520, "Text.TextColor"=u32 16711680) -> ()  [unwired: 1 in, 2 out]
              }
              frame 999 {
                n714 = for {
                  tunnel: w524 -> [w527] mode=indexing
                  n715 = call "Colour.vi"("result"="", "colourRef"=w527) -> ()  [unwired: 9 in, 1 out]
                }
                n716 = call "浮动通知2.vi"("通知内容"="请重新安装固定螺栓！" ("Status")) -> ()  [unwired: 11 in]
                n717 = shared-variable "我的电脑\\A17031611.lvlib\\设备状态2"(i16 31 ("设备状态")) -> ()  [unwired: 1 in, 1 out]
              }
              frame 1024 {
                n718 = global read "Global.vi" "ECU自动"() -> (w530:refnum<vi>)
                n719 = property class="Bool (严格)"(reference=w530, "Value"=FALSE) -> ()  [unwired: 1 in, 2 out]
              }
              frame 3721 {
                (unwired) "产品不合格程序锁定！" ("Status")
                n720 = local write "STEP3"("不合格锁定" ("STEP")) -> ()
              }
              frame 3722 {
                n721 = global read "Global.vi" "ECU自动"() -> (w533:refnum<vi>)
                n722 = property class="Bool (严格)"(reference=w533, "Value"=FALSE) -> ()  [unwired: 1 in, 2 out]
              }
              frame 3723 {
                (unwired) "请取出不合格产品并摆放至不合格品区！" ("Status")
              }
            }
          }
          frame "录入数据库" {
            n723 = stacked-sequence {
              frame #0 {
                n724 = Get Date/Time String(date format (0)=enum16{"short", "long", "abbreviated"}."short" ("日期格式(0)"), want seconds? (F)=FALSE ("需要秒？(F)")) -> (date string=w543:string, time string=w544:string)  [unwired: 1 in]
                n725 = global read "Global1.vi" "DEVICE_ID_ECU"() -> (w547:string)
                n726 = global read "Global1.vi" "CODE_ID_ECU"() -> (w546:string)
                n727 = global read "Global1.vi" "ECU工位生产结果"() -> (w538:string)
                n728 = global read "Global1.vi" "USER_ID"() -> (w545:string)
                n729 = Concatenate Strings(w543, " " ("字符串"), w544) -> (w539:string)
                n730 = Decimal String To Number(string=w547, default (0L)=i64 0 ("默认(0 I32)")) -> (number=w536:i64)  [unwired: 1 in, 1 out]
                n731 = Decimal String To Number(string=w545, default (0L)=i64 0 ("默认(0 I32)")) -> (number=w535:i64)  [unwired: 1 in, 1 out]
                n732 = Decimal String To Number(string=w546, default (0L)=i64 0 ("默认(0 I32)")) -> (number=w534:i64)  [unwired: 1 in, 1 out]
                n733 = global read "Global1.vi" "联机模式"() -> (w554:enum16{"单机", "联网"})
                n734 = Search and Replace String(replace all?=TRUE ("替换全部？(F)"), input string=w539, search string="/" ("替换字符串(\"\")"), replace string="-" ("替换字符串(\"\")")) -> (result string=w537:string)  [unwired: 4 in, 3 out]
                n735 = Bundle(w536, w535, w534, "ECU工位生产结果"=w538, "result string"=w537) -> (w560:T8)  [unwired: 1 in]
                n736 = call "GetSQLstring.vi"("联机模式"=w554) -> ("错误输出"=w557:errorcluster, "连接字符串"=w556:string)  [unwired: 9 in]
                n737 = Build Array(w560) -> (w561:T9)
                n738 = call-poly <vilib>:"DB Tools Open Connection.vi"("error in (no error)"=w557, "connection information"=w556) -> ("error out"=w555:errorcluster, "connection reference"=w558:T6)  [unwired: 6 in]
                n739 = for {
                  tunnel: w561 -> [w566] mode=indexing
                  tunnel: w558 -> [w564]
                  shift-right: [w562] -> w559
                  shift-left: w555 -> [w569]
                  w565 = string[] ["DEVICE_ID", "USER_ID", "CODE_ID", "RESULT_VALUE", "RESULT_TIME"] ("columns")
                  w567 = "Result" ("table")
                  n740 = call <vilib>:"DB Tools Insert Data.vi"("data"=w566, "error in (no error)"=w569, "columns"=w565, "table"=w567, "connection reference"=w564) -> ("error out"=w568:errorcluster, "connection reference out"=w563:T6)  [unwired: 5 in]
                  n741 = case shown="错误" w568 {
                    selector: w568 -> [w570 w591]
                    tunnel: w565 -> [_ w588]
                    tunnel: w563 -> [w571 w580]
                    tunnel: w567 -> [_ w592]
                    tunnel: w566 -> [_ w584]
                    tunnel: [w571 w579] -> _
                    tunnel: [w570 w578] -> w562
                    frame No Error {
                    }
                    frame Error {
                      n742 = Array Subset(array=w588, index=3 ("长度"), length=2 ("长度")) -> (w589:string[])
                      n743 = Unbundle(w584) -> (w573:i64, w576:i64, "ECU工位生产结果"=w583:string, "result string"=w582:string)  [unwired: 1 out]
                      n744 = Number To Decimal String(number=w576) -> (decimal integer string=w577:string)  [unwired: 1 in]
                      n745 = Number To Decimal String(number=w573) -> (decimal integer string=w572:string)  [unwired: 1 in]
                      n746 = Concatenate Strings("WHERE CODE_ID =" ("condition"), w577, "AND DEVICE_ID = ", w572) -> (w585:string)
                      n747 = Bundle("ECU工位生产结果"=w583, "result string"=w582) -> (w581:T10)  [unwired: 1 in]
                      n748 = call <vilib>:"Clear Errors.vi"("error in (no error)"=w591) -> ("error out"=w590:errorcluster)  [unwired: 5 in, 1 out]
                      n749 = call <vilib>:"DB Tools Update Data.vi"("condition"=w585, "data"=w581, "error in (no error)"=w590, "columns"=w589, "table"=w592, "connection reference"=w580) -> ("error out"=w578:errorcluster, "connection reference out"=w579:T6)  [unwired: 4 in]
                    }
                  }
                }
                n750 = call <vilib>:"Simple Error Handler.vi"("error in (no error)"=w559) -> ()  [unwired: 4 in, 5 out]
              }
              frame #1 {
                n751 = global read "Global1.vi" "CODE_ID_ECU"() -> (w594:string)
                n752 = global read "Global1.vi" "控制器码"() -> (w593:string)
                n753 = Format Into String(format string="UPDATE\ndbo.[Code]\nSET dbo.[Code].CODE_ECU = '%s'\n\nWHERE\ndbo.[Code].CODE_ID = %s\n" ("格式字符串"), w593, w594) -> (resulting string=w597:string)  [unwired: 2 in, 1 out]
                n754 = call "SQL_query.vi"("SQL query"=w597, "联机模式"=enum16{"单机", "联网"}."联网") -> ()  [unwired: 1 in, 3 out]
              }
              frame #2 {
              }
              frame #3 {
                n755 = call "浮动通知2.vi"("通知内容"="ECU工位数据录入成功！" ("Status")) -> ()  [unwired: 11 in]
                n756 = local write "STEP2"("等待" ("STEP2")) -> ()
                n757 = shared-variable "我的电脑\\A17031611.lvlib\\设备状态2"(i16 6 ("设备状态")) -> ()  [unwired: 1 in, 1 out]
              }
            }
          }
          frame "步骤" {
            n758 = case shown="\"控制器安装螺栓1\", 默认" "ECU步骤" {
              selector: "ECU步骤" -> [w604 _]
              tunnel: [w603 "等待"] -> w601
              frame "控制器安装螺栓1", Default {
                n759 = global read "Global.vi" "控制器安装支架"() -> (w606:bool[])
                n760 = Index Array(array=w606, index=w604) -> (element=w605:bool)
                n761 = case shown="真" w605 {
                  tunnel: w604 -> [_ w611]
                  tunnel: ["步骤" w610] -> w603
                  frame False {
                    n762 = local read "ECU步骤"() -> (w609:T2)
                    n763 = Increment(x=w609) -> (x+1=w608:T2)
                    n764 = local write "ECU步骤"(w608) -> ()
                  }
                  frame True {
                    n765 = case shown="\"安装线卡轧带\"" w611 {
                      tunnel: ["等待" "等待" "等待" "等待" "等待" "等待" "等待" "等待" "等待"] -> w610
                      frame "控制器安装螺栓1", Default {
                        n766 = shared-variable "我的电脑\\A17031611.lvlib\\设备状态2"(i16 31 ("设备状态控制字")) -> ()  [unwired: 1 in, 1 out]
                      }
                      frame "控制器安装螺栓2" {
                        n767 = shared-variable "我的电脑\\A17031611.lvlib\\设备状态2"(i16 33 ("设备状态控制字")) -> ()  [unwired: 1 in, 1 out]
                      }
                      frame "控制器安装螺栓3" {
                        n768 = shared-variable "我的电脑\\A17031611.lvlib\\设备状态2"(i16 35 ("设备状态控制字")) -> ()  [unwired: 1 in, 1 out]
                      }
                      frame "安装支架螺栓1" {
                        n769 = shared-variable "我的电脑\\A17031611.lvlib\\设备状态2"(i16 41 ("设备状态控制字")) -> ()  [unwired: 1 in, 1 out]
                      }
                      frame "安装支架螺栓2" {
                        n770 = shared-variable "我的电脑\\A17031611.lvlib\\设备状态2"(i16 43 ("设备状态控制字")) -> ()  [unwired: 1 in, 1 out]
                      }
                      frame "安装支架螺栓3" {
                        n771 = shared-variable "我的电脑\\A17031611.lvlib\\设备状态2"(i16 45 ("设备状态控制字")) -> ()  [unwired: 1 in, 1 out]
                      }
                      frame "安装支架螺栓4" {
                        n772 = shared-variable "我的电脑\\A17031611.lvlib\\设备状态2"(i16 47 ("设备状态控制字")) -> ()  [unwired: 1 in, 1 out]
                      }
                      frame "涂色标" {
                        n773 = shared-variable "我的电脑\\A17031611.lvlib\\设备状态2"(i16 60 ("设备状态控制字")) -> ()  [unwired: 1 in, 1 out]
                      }
                      frame "安装线卡轧带" {
                        n774 = shared-variable "我的电脑\\A17031611.lvlib\\设备状态2"(i16 70 ("设备状态控制字")) -> ()  [unwired: 1 in, 1 out]
                      }
                    }
                  }
                }
              }
              frame "完成" {
                n775 = shared-variable "我的电脑\\A17031611.lvlib\\设备状态2"(i16 81 ("设备状态控制字")) -> ()  [unwired: 1 in, 1 out]
              }
            }
            n776 = local write "STEP2"(w601) -> ()
          }
        }
        n777 = case shown="\"初始化\"" "STEP1" {
          frame "等待", Default {
            n778 = local write "STEP1"("自动" ("STEP1")) -> ()
            n779 = Wait (ms)(milliseconds to wait=u32 200 ("等待时间（毫秒）")) -> ()  [unwired: 1 out]
          }
          frame "初始化" {
            n780 = local write "STEP1"("步骤" ("STEP")) -> ()
            n781 = local write "控制器支架"(T1."控制器支架螺栓1" ("控制器支架")) -> ()
          }
          frame "自动" {
            # "5=31\n4=32\n3=33\n2=34\n1=35"
            n782 = shared-variable "我的电脑\\A17031611.lvlib\\控制器支架螺栓数量"() -> (w58:i16)  [unwired: 1 in, 1 out]
            n783 = shared-variable "我的电脑\\A17031611.lvlib\\设备状态1"() -> (w59:i16)  [unwired: 1 in, 1 out]
            n784 = global read "A170316-11.vi" "控制器支架LED"() -> (w60:refnum<vi>[])
            n785 = case shown="10" w59 {
              tunnel: w60 -> [_ _ _ _ _ _ _ _ _ _ _ _ _ w105 _ w115 w122 w138]
              tunnel: w58 -> [_ _ _ _ _ _ _ _ _ _ _ _ _ _ _ _ _ _]
              frame 0, Default {
              }
              frame 10 {
                n786 = local write "STEP1"("初始化" ("STEP1")) -> ()
              }
              frame 30 {
                n787 = control-ref of="控制器支架螺栓1拧紧确认"() -> (w63:refnum<vi>)
                n788 = call "Colour.vi"("result"="等待", "colourRef"=w63) -> ()  [unwired: 9 in, 1 out]
                n789 = call "浮动通知2.vi"("通知内容"="请安装第一颗螺丝并拧紧！" ("Status")) -> ()  [unwired: 11 in]
              }
              frame 31 {
                n790 = flat-sequence {
                  frame #0 {
                    n791 = control-ref of="控制器支架螺栓1拧紧确认"() -> (w66:refnum<vi>)
                    n792 = call "Colour.vi"("result"="OK", "colourRef"=w66) -> ()  [unwired: 9 in, 1 out]
                  }
                  frame #1 {
                    n793 = local read "控制器支架"() -> (w69:T1)
                    n794 = Increment(x=w69) -> (x+1=w68:T1)
                    n795 = local write "STEP1"("步骤" ("STEP1")) -> ()
                    n796 = local write "控制器支架"(w68) -> ()
                  }
                }
              }
              frame 32 {
                n797 = control-ref of="控制器支架螺栓2拧紧确认"() -> (w71:refnum<vi>)
                n798 = call "Colour.vi"("result"="等待", "colourRef"=w71) -> ()  [unwired: 9 in, 1 out]
                n799 = call "浮动通知2.vi"("通知内容"="请安装第二颗螺丝并拧紧！" ("Status")) -> ()  [unwired: 11 in]
              }
              frame 33 {
                n800 = flat-sequence {
                  frame #0 {
                    n801 = control-ref of="控制器支架螺栓2拧紧确认"() -> (w73:refnum<vi>)
                    n802 = call "Colour.vi"("result"="OK", "colourRef"=w73) -> ()  [unwired: 9 in, 1 out]
                  }
                  frame #1 {
                    n803 = local read "控制器支架"() -> (w76:T1)
                    n804 = Increment(x=w76) -> (x+1=w75:T1)
                    n805 = local write "控制器支架"(w75) -> ()
                    n806 = local write "STEP1"("步骤" ("STEP1")) -> ()
                  }
                }
              }
              frame 34 {
                # "控制器支架螺栓1"
                n807 = control-ref of="控制器支架螺栓3拧紧确认"() -> (w78:refnum<vi>)
                n808 = call "Colour.vi"("result"="等待", "colourRef"=w78) -> ()  [unwired: 9 in, 1 out]
                n809 = call "浮动通知2.vi"("通知内容"="请安装第三颗螺丝并拧紧！" ("Status")) -> ()  [unwired: 11 in]
              }
              frame 35 {
                n810 = flat-sequence {
                  frame #0 {
                    n811 = control-ref of="控制器支架螺栓3拧紧确认"() -> (w81:refnum<vi>)
                    n812 = call "Colour.vi"("result"="OK", "colourRef"=w81) -> ()  [unwired: 9 in, 1 out]
                  }
                  frame #1 {
                    n813 = local read "控制器支架"() -> (w84:T1)
                    n814 = Increment(x=w84) -> (x+1=w83:T1)
                    n815 = local write "控制器支架"(w83) -> ()
                    n816 = local write "STEP1"("步骤" ("STEP1")) -> ()
                  }
                }
              }
              frame 36 {
                n817 = control-ref of="控制器支架螺栓4拧紧确认"() -> (w86:refnum<vi>)
                n818 = call "浮动通知2.vi"("通知内容"="请安装第四颗螺丝并拧紧！" ("Status")) -> ()  [unwired: 11 in]
                n819 = call "Colour.vi"("result"="等待", "colourRef"=w86) -> ()  [unwired: 9 in, 1 out]
              }
              frame 37 {
                n820 = flat-sequence {
                  frame #0 {
                    n821 = control-ref of="控制器支架螺栓4拧紧确认"() -> (w89:refnum<vi>)
                    n822 = call "Colour.vi"("result"="OK", "colourRef"=w89) -> ()  [unwired: 9 in, 1 out]
                  }
                  frame #1 {
                    n823 = local read "控制器支架"() -> (w92:T1)
                    n824 = Increment(x=w92) -> (x+1=w91:T1)
                    n825 = local write "控制器支架"(w91) -> ()
                    n826 = local write "STEP1"("步骤" ("STEP1")) -> ()
                  }
                }
              }
              frame 38 {
                n827 = control-ref of="控制器支架螺栓5拧紧确认"() -> (w94:refnum<vi>)
                n828 = call "Colour.vi"("result"="等待", "colourRef"=w94) -> ()  [unwired: 9 in, 1 out]
                n829 = call "浮动通知2.vi"("通知内容"="请安装第五颗螺丝并拧紧！" ("Status")) -> ()  [unwired: 11 in]
              }
              frame 39 {
                n830 = flat-sequence {
                  frame #0 {
                    n831 = control-ref of="控制器支架螺栓5拧紧确认"() -> (w97:refnum<vi>)
                    n832 = call "Colour.vi"("result"="OK", "colourRef"=w97) -> ()  [unwired: 9 in, 1 out]
                  }
                  frame #1 {
                    n833 = local read "控制器支架"() -> (w100:T1)
                    n834 = Increment(x=w100) -> (x+1=w99:T1)
                    n835 = local write "控制器支架"(w99) -> ()
                    n836 = local write "STEP1"("步骤" ("STEP1")) -> ()
                  }
                }
              }
              frame 60 {
                n837 = control-ref of="控制器支架涂色标"() -> (w102:refnum<vi>)
                n838 = call "Colour.vi"("result"="等待", "colourRef"=w102) -> ()  [unwired: 9 in, 1 out]
                n839 = call "浮动通知2.vi"("通知内容"="请控制器固定螺栓涂色标！" ("Status")) -> ()  [unwired: 11 in]
              }
              frame 61 {
                n840 = Index Array(array=w105, index #1=4 ("索引")) -> ()  [unwired: 1 in, 2 out]
                n841 = flat-sequence {
                  frame #0 {
                    n842 = control-ref of="控制器支架涂色标"() -> (w108:refnum<vi>)
                    n843 = call "Colour.vi"("result"="OK", "colourRef"=w108) -> ()  [unwired: 9 in, 1 out]
                  }
                  frame #1 {
                    n844 = local read "控制器支架"() -> (w111:T1)
                    n845 = Increment(x=w111) -> (x+1=w110:T1)
                    n846 = local write "控制器支架"(w110) -> ()
                    n847 = local write "STEP1"("步骤" ("STEP1")) -> ()
                  }
                }
              }
              frame 70 {
                n848 = control-ref of="控制器支架安装线卡扎带"() -> (w112:refnum<vi>)
                n849 = call "Colour.vi"("result"="等待", "colourRef"=w112) -> ()  [unwired: 9 in, 1 out]
                n850 = call "浮动通知2.vi"("通知内容"="请安装轧带并取走工件！" ("Status")) -> ()  [unwired: 11 in]
              }
              frame 81 {
                n851 = Index Array(array=w115, index=6 ("索引")) -> ()  [unwired: 1 out]
                n852 = flat-sequence {
                  frame #0 {
                    n853 = control-ref of="控制器支架安装线卡扎带"() -> (w118:refnum<vi>)
                    n854 = call "Colour.vi"("result"="OK", "colourRef"=w118) -> ()  [unwired: 9 in, 1 out]
                  }
                  frame #1 {
                    n855 = local read "控制器支架"() -> (w121:T1)
                    n856 = Increment(x=w121) -> (x+1=w120:T1)
                    n857 = local write "控制器支架"(w120) -> ()
                    n858 = local write "STEP1"("步骤" ("STEP1")) -> ()
                  }
                }
              }
              frame 91 {
                n859 = for {
                  tunnel: w122 -> [w126] mode=indexing
                  n860 = call "Colour.vi"("result"="", "colourRef"=w126) -> ()  [unwired: 9 in, 1 out]
                }
                n861 = shared-variable "我的电脑\\A17031611.lvlib\\设备状态1"(i16 10 ("设备状态")) -> ()  [unwired: 1 in, 1 out]
                n862 = local write "STEP1"("初始化" ("STEP1")) -> ()
                n863 = call "浮动通知2.vi"("通知内容"="控制器和支架合装完成！" ("Status")) -> ()  [unwired: 11 in]
              }
              frame 999 {
                n864 = Index Array(array=w138, index #1=0 ("索引")) -> (element #1=w141:refnum<vi>, element #2=w135:refnum<vi>, element #3=w133:refnum<vi>, element #4=w131:refnum<vi>, element #5=w128:refnum<vi>)  [unwired: 4 in]
                n865 = call "Colour.vi"("result"="", "colourRef"=w128) -> ()  [unwired: 9 in, 1 out]
                n866 = call "Colour.vi"("result"="", "colourRef"=w135) -> ()  [unwired: 9 in, 1 out]
                n867 = call "Colour.vi"("result"="", "colourRef"=w133) -> ()  [unwired: 9 in, 1 out]
                n868 = call "Colour.vi"("result"="", "colourRef"=w131) -> ()  [unwired: 9 in, 1 out]
                n869 = call "Colour.vi"("result"="NG", "colourRef"=w141) -> ()  [unwired: 9 in, 1 out]
                n870 = call "浮动通知2.vi"("通知内容"="安装固定螺栓未完成，请重新安装！" ("Status")) -> ()  [unwired: 11 in]
                n871 = shared-variable "我的电脑\\A17031611.lvlib\\设备状态1"(i16 10 ("设备状态")) -> ()  [unwired: 1 in, 1 out]
              }
            }
          }
          frame "步骤" {
            n872 = case shown="\"控制器支架螺栓1\", 默认" "控制器支架" {
              selector: "控制器支架" -> [w145 _]
              tunnel: [w144 "自动"] -> w142
              frame "控制器支架螺栓1", Default {
                n873 = global read "Global.vi" "控制器支架"() -> (w147:bool[])
                n874 = Index Array(array=w147, index=w145) -> (element=w146:bool)
                n875 = case shown="真" w146 {
                  tunnel: w145 -> [_ w152]
                  tunnel: ["步骤" w151] -> w144
                  frame False {
                    n876 = local read "控制器支架"() -> (w150:T1)
                    n877 = Increment(x=w150) -> (x+1=w149:T1)
                    n878 = local write "控制器支架"(w149) -> ()
                  }
                  frame True {
                    n879 = case shown="\"安装线卡轧带\"" w152 {
                      tunnel: ["等待" "等待" "等待" "等待" "等待" "等待" "等待"] -> w151
                      frame "控制器支架螺栓1", Default {
                        n880 = shared-variable "我的电脑\\A17031611.lvlib\\设备状态1"(i16 30 ("设备状态1")) -> ()  [unwired: 1 in, 1 out]
                      }
                      frame "控制器支架螺栓2" {
                        n881 = shared-variable "我的电脑\\A17031611.lvlib\\设备状态1"(i16 32 ("设备状态1")) -> ()  [unwired: 1 in, 1 out]
                      }
                      frame "控制器支架螺栓3" {
                        n882 = shared-variable "我的电脑\\A17031611.lvlib\\设备状态1"(i16 34 ("设备状态1")) -> ()  [unwired: 1 in, 1 out]
                      }
                      frame "控制器支架螺栓4" {
                        n883 = shared-variable "我的电脑\\A17031611.lvlib\\设备状态1"(i16 36 ("设备状态1")) -> ()  [unwired: 1 in, 1 out]
                      }
                      frame "控制器支架螺栓5" {
                        n884 = shared-variable "我的电脑\\A17031611.lvlib\\设备状态1"(i16 38 ("设备状态1")) -> ()  [unwired: 1 in, 1 out]
                      }
                      frame "涂色标" {
                        n885 = shared-variable "我的电脑\\A17031611.lvlib\\设备状态1"(i16 60 ("设备状态1")) -> ()  [unwired: 1 in, 1 out]
                      }
                      frame "安装线卡轧带" {
                        n886 = shared-variable "我的电脑\\A17031611.lvlib\\设备状态1"(i16 70 ("设备状态1")) -> ()  [unwired: 1 in, 1 out]
                      }
                    }
                  }
                }
              }
              frame "完成" {
                n887 = shared-variable "我的电脑\\A17031611.lvlib\\设备状态1"(i16 91 ("设备状态")) -> ()  [unwired: 1 in, 1 out]
              }
            }
            n888 = local write "STEP1"(w142) -> ()
          }
        }
        n889 = global read "Global.vi" "程序关闭"() -> (w53:bool)
      }
      n890 = while {
        stop <- w1149 stop-if-true
        n891 = global read "Global.vi" "产品型号"() -> (w1150:string)
        n892 = Wait Until Next ms Multiple(millisecond multiple=u32 5 ("毫秒倍数")) -> ()  [unwired: 1 out]
        n893 = call "Is Value Changed.vim"("value"=w1150) -> ("changed or first call?"=w1151:bool)
        n894 = event shown="[2] \"更换产品\": 值改变" {
          selector: _ -> [_ _ _ _]
          dyn-events: _ -> [_ _ _ _]
          timeout: 5 -> [_ _ _ _]
          tunnel: w1150 -> [_ w1170 w1457 _]
          event Timeout {
            n895 = event-data() -> ()  [unwired: 1 in, 3 out]
            n896 = shared-variable "我的电脑\\A17031611.lvlib\\错误代码"() -> (w1154:u16)  [unwired: 1 in, 1 out]
            n897 = feedback #1() -> (w1164:u16)  [unwired: 1 in]
            n898 = feedback-in #1(w1154) -> ()
            n899 = Greater Or Equal?(x=w1154, y=i16 5000) -> (x >= y?=w1162:bool)
            n900 = Less?(x=w1154, y=i16 5200) -> (x < y?=w1163:bool)
            n901 = Equal?(x=w1154, y=w1164) -> (x = y?=w1161:bool)
            n902 = global read "Global.vi" "报警图标"() -> (w1156:refnum<vi>)
            n903 = And(x=w1162, y=w1163) -> (x .and. y?=w1155:bool)
            n904 = property class="Bool"(reference=w1156, "Value"=w1155) -> ()  [unwired: 1 in, 2 out]
            n905 = Bundle By Name(cluster=errorcluster {"status"=FALSE, "code"=0, "source"=""} ("错误常量"), "status"=w1155, "code"=w1154) -> (w1160:errorcluster)
            n906 = case shown="真" w1161 {
              tunnel: w1160 -> [w1169 _]
              frame False {
                n907 = call "报警处理.vi"("错误常量"=w1169) -> ()  [unwired: 9 in, 2 out]
              }
              frame True {
              }
            }
            n908 = case shown="0" w1154 {
              frame 0 {
                n909 = global read "Global.vi" "报警图标"() -> (w1165:refnum<vi>)
                n910 = property class="Bool"(reference=w1165, "Visible"=FALSE ("可见")) -> ()  [unwired: 1 in, 2 out]
              }
              frame 1, Default {
                n911 = global read "Global.vi" "报警图标"() -> (w1168:refnum<vi>)
                n912 = property class="Bool"(reference=w1168, "Visible"=TRUE ("可见")) -> ()  [unwired: 1 in, 2 out]
              }
            }
          }
          event "前序OK？": Value Change {
            n913 = event-data() -> ()  [unwired: 1 in, 6 out]
            n914 = stacked-sequence {
              tunnel: w1170 -> [_ w1224]
              frame #0 {
                n915 = disable-structure shown="禁用" {
                  frame Disabled {
                    n916 = control-ref of="安装扎带并取走工件"() -> (w1177:refnum<vi>)
                    n917 = control-ref of="安装扎带和线卡并取走工件"() -> (w1176:refnum<vi>)
                    n918 = control-ref of="控制器安装螺栓1拧紧确认"() -> (w1197:refnum<vi>)
                    n919 = control-ref of="控制器安装螺栓2拧紧确认"() -> (w1194:refnum<vi>)
                    n920 = control-ref of="安装支架涂色标"() -> (w1196:refnum<vi>)
                    n921 = control-ref of="安装支架扎带安装"() -> (w1180:refnum<vi>)
                    n922 = control-ref of="安装支架线卡扎带安装"() -> (w1179:refnum<vi>)
                    n923 = control-ref of="控制器安装螺栓3拧紧确认"() -> (w1175:refnum<vi>)
                    n924 = control-ref of="安装支架螺栓1拧紧确认"() -> (w1199:refnum<vi>)
                    n925 = control-ref of="安装支架螺栓4拧紧确认"() -> (w1171:refnum<vi>)
                    n926 = control-ref of="安装弹性垫圈弹簧并按启动拍照"() -> (w1186:refnum<vi>)
                    n927 = control-ref of="安装扎带并取走工件"() -> (w1181:refnum<vi>)
                    n928 = control-ref of="电机安装螺栓2扭矩确认"() -> (w1184:refnum<vi>)
                    n929 = control-ref of="安装支架螺栓3拧紧确认"() -> (w1174:refnum<vi>)
                    n930 = control-ref of="安装支架螺栓2拧紧确认"() -> (w1198:refnum<vi>)
                    n931 = control-ref of="电机安装螺栓3扭矩确认"() -> (w1172:refnum<vi>)
                    n932 = control-ref of="按启动按钮拍照确认"() -> (w1183:refnum<vi>)
                    n933 = control-ref of="电机安装螺栓1扭矩确认"() -> (w1185:refnum<vi>)
                    n934 = control-ref of="控制器支架涂色标"() -> (w1188:refnum<vi>)
                    n935 = control-ref of="涂色标"() -> (w1182:refnum<vi>)
                    n936 = Build Array(w1199, w1198, w1197, w1194, w1196, w1180, w1179, w1175, w1174, w1171) -> (w1195:refnum<vi>[])
                    n937 = control-ref of="控制器支架螺栓1拧紧确认"() -> (w1192:refnum<vi>)
                    n938 = control-ref of="控制器支架螺栓3拧紧确认"() -> (w1190:refnum<vi>)
                    n939 = for {
                      tunnel: w1195 -> [w1223] mode=indexing
                      i -> [w1222]
                      n940 = Multiply(x=60, y=w1222) -> (x*y=w1217:i32)
                      n941 = Add(x=340 ("y"), y=w1217) -> (x+y=w1219:i32)
                      n942 = Bundle("y"=-500, w1219) -> (w1218:cluster{"y":i32, i32})  [unwired: 1 in]
                      n943 = property class="Bool (严格)"(reference=w1223, "Position"=w1218) -> ()  [unwired: 1 in, 2 out]
                    }
                    n944 = control-ref of="控制器支架安装线卡扎带"() -> (w1178:refnum<vi>)
                    n945 = control-ref of="控制器支架螺栓4拧紧确认"() -> (w1189:refnum<vi>)
                    n946 = Build Array(w1186, w1185, w1184, w1183, w1182, w1181, w1177, w1176, w1172) -> (w1187:refnum<vi>[])
                    n947 = control-ref of="控制器支架螺栓2拧紧确认"() -> (w1191:refnum<vi>)
                    n948 = control-ref of="控制器支架螺栓5拧紧确认"() -> (w1173:refnum<vi>)
                    n949 = for {
                      tunnel: w1187 -> [w1207] mode=indexing
                      i -> [w1206]
                      n950 = Multiply(x=60, y=w1206) -> (x*y=w1204:i32)
                      n951 = Add(x=w1204, y=340) -> (x+y=w1201:i32)
                      n952 = Bundle("y"=-1500, w1201) -> (w1200:cluster{"y":i32, i32})  [unwired: 1 in]
                      n953 = property class="Bool (严格)"(reference=w1207, "Position"=w1200) -> ()  [unwired: 1 in, 2 out]
                    }
                    n954 = Build Array(w1192, w1191, w1190, w1189, w1188, w1178, w1173) -> (w1193:refnum<vi>[])
                    n955 = for {
                      tunnel: w1193 -> [w1215] mode=indexing
                      i -> [w1214]
                      n956 = Multiply(x=60, y=w1214) -> (x*y=w1212:i32)
                      n957 = Add(x=w1212, y=345) -> (x+y=w1209:i32)
                      n958 = Bundle("y"=-1000, w1209) -> (w1208:cluster{"y":i32, i32})  [unwired: 1 in]
                      n959 = property class="Bool (严格)"(reference=w1215, "Position"=w1208) -> ()  [unwired: 1 in, 2 out]
                    }
                  }
                  frame Enabled {
                  }
                }
              }
              frame #1 {
                n960 = disable-structure shown="禁用" {
                  disable-tunnel: w1224 -> [w1225 _]
                  frame Disabled {
                    n961 = case shown="\"R092B\"" w1225 {
                      frame Default {
                      }
                      frame "R92A" {
                        n962 = control-ref of="控制器安装螺栓2拧紧确认"() -> (w1230:refnum<vi>)
                        n963 = control-ref of="安装支架螺栓4拧紧确认"() -> (w1232:refnum<vi>)
                        n964 = control-ref of="控制器安装螺栓1拧紧确认"() -> (w1231:refnum<vi>)
                        n965 = control-ref of="安装支架螺栓1拧紧确认"() -> (w1235:refnum<vi>)
                        n966 = control-ref of="安装支架螺栓3拧紧确认"() -> (w1233:refnum<vi>)
                        n967 = control-ref of="控制器安装螺栓3拧紧确认"() -> (w1229:refnum<vi>)
                        n968 = control-ref of="安装支架涂色标"() -> (w1228:refnum<vi>)
                        n969 = control-ref of="安装支架螺栓2拧紧确认"() -> (w1234:refnum<vi>)
                        n970 = control-ref of="安装弹性垫圈弹簧并按启动拍照"() -> (w1242:refnum<vi>)
                        n971 = control-ref of="电机安装螺栓3扭矩确认"() -> (w1236:refnum<vi>)
                        n972 = control-ref of="电机安装螺栓1扭矩确认"() -> (w1241:refnum<vi>)
                        n973 = control-ref of="电机安装螺栓2扭矩确认"() -> (w1240:refnum<vi>)
                        n974 = control-ref of="按启动按钮拍照确认"() -> (w1239:refnum<vi>)
                        n975 = control-ref of="安装扎带并取走工件"() -> (w1237:refnum<vi>)
                        n976 = Build Array(w1235, w1234, w1233, w1232, w1231, w1230, w1229, w1228) -> (w1227:refnum<vi>[])
                        n977 = control-ref of="涂色标"() -> (w1238:refnum<vi>)
                        n978 = for {
                          tunnel: w1227 -> [w1272] mode=indexing
                          i -> [w1271]
                          n979 = Multiply(x=60, y=w1271) -> (x*y=w1266:i32)
                          n980 = Add(x=340 ("y"), y=w1266) -> (x+y=w1268:i32)
                          n981 = Bundle("y"=1775, w1268) -> (w1267:cluster{"y":i32, i32})  [unwired: 1 in]
                          n982 = property class="Bool (严格)"(reference=w1272, "Position"=w1267) -> ()  [unwired: 1 in, 2 out]
                        }
                        n983 = Build Array(w1242, w1241, w1240, w1236, w1239, w1238, w1237) -> (w1243:refnum<vi>[])
                        n984 = control-ref of="控制器支架螺栓2拧紧确认"() -> (w1246:refnum<vi>)
                        n985 = control-ref of="控制器支架螺栓1拧紧确认"() -> (w1247:refnum<vi>)
                        n986 = control-ref of="控制器支架螺栓3拧紧确认"() -> (w1245:refnum<vi>)
                        n987 = control-ref of="控制器支架螺栓4拧紧确认"() -> (w1244:refnum<vi>)
                        n988 = control-ref of="控制器支架涂色标"() -> (w1226:refnum<vi>)
                        n989 = for {
                          tunnel: w1243 -> [w1256] mode=indexing
                          i -> [w1255]
                          n990 = Multiply(x=60, y=w1255) -> (x*y=w1253:i32)
                          n991 = Add(x=w1253, y=340) -> (x+y=w1250:i32)
                          n992 = Bundle("y"=2115, w1250) -> (w1249:cluster{"y":i32, i32})  [unwired: 1 in]
                          n993 = property class="Bool (严格)"(reference=w1256, "Position"=w1249) -> ()  [unwired: 1 in, 2 out]
                        }
                        n994 = Build Array(w1247, w1246, w1245, w1244, w1226) -> (w1248:refnum<vi>[])
                        n995 = for {
                          tunnel: w1248 -> [w1264] mode=indexing
                          i -> [w1263]
                          n996 = Multiply(x=60, y=w1263) -> (x*y=w1261:i32)
                          n997 = Add(x=w1261, y=345) -> (x+y=w1258:i32)
                          n998 = Bundle("y"=1445, w1258) -> (w1257:cluster{"y":i32, i32})  [unwired: 1 in]
                          n999 = property class="Bool (严格)"(reference=w1264, "Position"=w1257) -> ()  [unwired: 1 in, 2 out]
                        }
                      }
                      frame "R128" {
                        # "1345"
                        n1000 = control-ref of="安装支架螺栓2拧紧确认"() -> (w1288:refnum<vi>)
                        n1001 = control-ref of="安装支架涂色标"() -> (w1287:refnum<vi>)
                        n1002 = control-ref of="安装支架螺栓1拧紧确认"() -> (w1289:refnum<vi>)
                        n1003 = control-ref of="控制器安装螺栓1拧紧确认"() -> (w1291:refnum<vi>)
                        n1004 = control-ref of="控制器安装螺栓2拧紧确认"() -> (w1290:refnum<vi>)
                        n1005 = control-ref of="安装弹性垫圈弹簧并按启动拍照"() -> (w1282:refnum<vi>)
                        n1006 = control-ref of="电机安装螺栓1扭矩确认"() -> (w1281:refnum<vi>)
                        n1007 = control-ref of="电机安装螺栓2扭矩确认"() -> (w1280:refnum<vi>)
                        n1008 = control-ref of="涂色标"() -> (w1278:refnum<vi>)
                        n1009 = control-ref of="安装扎带并取走工件"() -> (w1277:refnum<vi>)
                        n1010 = control-ref of="按启动按钮拍照确认"() -> (w1279:refnum<vi>)
                        n1011 = Build Array(w1291, w1290, w1289, w1288, w1287) -> (w1294:refnum<vi>[])
                        n1012 = control-ref of="控制器支架螺栓2拧紧确认"() -> (w1285:refnum<vi>)
                        n1013 = control-ref of="控制器支架螺栓1拧紧确认"() -> (w1286:refnum<vi>)
                        n1014 = control-ref of="控制器支架螺栓3拧紧确认"() -> (w1284:refnum<vi>)
                        n1015 = control-ref of="控制器支架螺栓5拧紧确认"() -> ()  [unwired: 1 out]
                        n1016 = control-ref of="控制器支架涂色标"() -> (w1276:refnum<vi>)
                        n1017 = control-ref of="控制器支架螺栓4拧紧确认"() -> (w1283:refnum<vi>)
                        n1018 = for {
                          tunnel: w1294 -> [w1326] mode=indexing
                          i -> [w1325]
                          n1019 = Multiply(x=60, y=w1325) -> (x*y=w1320:i32)
                          n1020 = Add(x=438 ("y"), y=w1320) -> (x+y=w1322:i32)
                          n1021 = Bundle("y"=-1495, w1322) -> (w1321:cluster{"y":i32, i32})  [unwired: 1 in]
                          n1022 = property class="Bool (严格)"(reference=w1326, "Position"=w1321) -> ()  [unwired: 1 in, 2 out]
                        }
                        n1023 = Build Array(w1282, w1281, w1280, w1279, w1278, w1277) -> (w1292:refnum<vi>[])
                        n1024 = for {
                          tunnel: w1292 -> [w1310] mode=indexing
                          i -> [w1309]
                          n1025 = Multiply(x=60, y=w1309) -> (x*y=w1307:i32)
                          n1026 = Add(x=w1307, y=438) -> (x+y=w1304:i32)
                          n1027 = Bundle("y"=-1145, w1304) -> (w1303:cluster{"y":i32, i32})  [unwired: 1 in]
                          n1028 = property class="Bool (严格)"(reference=w1310, "Position"=w1303) -> ()  [unwired: 1 in, 2 out]
                        }
                        n1029 = control-ref of="安装支架螺栓3拧紧确认"() -> (w1275:refnum<vi>)
                        n1030 = Build Array(w1286, w1285, w1284, w1283, w1276) -> (w1293:refnum<vi>[])
                        n1031 = control-ref of="安装支架螺栓4拧紧确认"() -> (w1273:refnum<vi>)
                        n1032 = for {
                          tunnel: w1293 -> [w1318] mode=indexing
                          i -> [w1317]
                          n1033 = Multiply(x=60, y=w1317) -> (x*y=w1315:i32)
                          n1034 = Add(x=w1315, y=438) -> (x+y=w1312:i32)
                          n1035 = Bundle("y"=-1820, w1312) -> (w1311:cluster{"y":i32, i32})  [unwired: 1 in]
                          n1036 = property class="Bool (严格)"(reference=w1318, "Position"=w1311) -> ()  [unwired: 1 in, 2 out]
                        }
                        n1037 = Build Array(w1275, w1273) -> (w1274:refnum<vi>[])
                        n1038 = for {
                          tunnel: w1274 -> [w1302] mode=indexing
                          i -> [w1301]
                          n1039 = Multiply(x=60, y=w1301) -> (x*y=w1299:i32)
                          n1040 = Add(x=w1299, y=438) -> (x+y=w1296:i32)
                          n1041 = Bundle("y"=-100, w1296) -> (w1295:cluster{"y":i32, i32})  [unwired: 1 in]
                          n1042 = property class="Bool (严格)"(reference=w1302, "Position"=w1295) -> ()  [unwired: 1 in, 2 out]
                        }
                      }
                      frame "R092B" {
                        # "1345"
                        n1043 = control-ref of="安装支架螺栓3拧紧确认"() -> (w1327:refnum<vi>)
                        n1044 = control-ref of="安装支架涂色标"() -> (w1339:refnum<vi>)
                        n1045 = control-ref of="安装支架螺栓2拧紧确认"() -> (w1340:refnum<vi>)
                        n1046 = control-ref of="安装支架螺栓1拧紧确认"() -> (w1341:refnum<vi>)
                        n1047 = control-ref of="控制器安装螺栓1拧紧确认"() -> (w1343:refnum<vi>)
                        n1048 = control-ref of="控制器安装螺栓2拧紧确认"() -> (w1342:refnum<vi>)
                        n1049 = control-ref of="安装弹性垫圈弹簧并按启动拍照"() -> (w1334:refnum<vi>)
                        n1050 = control-ref of="电机安装螺栓1扭矩确认"() -> (w1333:refnum<vi>)
                        n1051 = control-ref of="电机安装螺栓2扭矩确认"() -> (w1332:refnum<vi>)
                        n1052 = control-ref of="涂色标"() -> (w1330:refnum<vi>)
                        n1053 = control-ref of="安装扎带并取走工件"() -> (w1329:refnum<vi>)
                        n1054 = control-ref of="按启动按钮拍照确认"() -> (w1331:refnum<vi>)
                        n1055 = Build Array(w1343, w1342, w1341, w1340, w1327, w1339) -> (w1346:refnum<vi>[])
                        n1056 = control-ref of="控制器支架螺栓2拧紧确认"() -> (w1337:refnum<vi>)
                        n1057 = control-ref of="控制器支架螺栓1拧紧确认"() -> (w1338:refnum<vi>)
                        n1058 = control-ref of="控制器支架螺栓3拧紧确认"() -> (w1336:refnum<vi>)
                        n1059 = control-ref of="控制器支架涂色标"() -> (w1328:refnum<vi>)
                        n1060 = control-ref of="控制器支架螺栓4拧紧确认"() -> (w1335:refnum<vi>)
                        n1061 = for {
                          tunnel: w1346 -> [w1370] mode=indexing
                          i -> [w1369]
                          n1062 = Multiply(x=60, y=w1369) -> (x*y=w1364:i32)
                          n1063 = Add(x=438 ("y"), y=w1364) -> (x+y=w1366:i32)
                          n1064 = Bundle("y"=-1495, w1366) -> (w1365:cluster{"y":i32, i32})  [unwired: 1 in]
                          n1065 = property class="Bool (严格)"(reference=w1370, "Position"=w1365) -> ()  [unwired: 1 in, 2 out]
                        }
                        n1066 = Build Array(w1334, w1333, w1332, w1331, w1330, w1329) -> (w1344:refnum<vi>[])
                        n1067 = for {
                          tunnel: w1344 -> [w1354] mode=indexing
                          i -> [w1353]
                          n1068 = Multiply(x=60, y=w1353) -> (x*y=w1351:i32)
                          n1069 = Add(x=w1351, y=438) -> (x+y=w1348:i32)
                          n1070 = Bundle("y"=-1145, w1348) -> (w1347:cluster{"y":i32, i32})  [unwired: 1 in]
                          n1071 = property class="Bool (严格)"(reference=w1354, "Position"=w1347) -> ()  [unwired: 1 in, 2 out]
                        }
                        n1072 = Build Array(w1338, w1337, w1336, w1335, w1328) -> (w1345:refnum<vi>[])
                        n1073 = control-ref of="控制器支架螺栓5拧紧确认"() -> ()  [unwired: 1 out]
                        n1074 = for {
                          tunnel: w1345 -> [w1362] mode=indexing
                          i -> [w1361]
                          n1075 = Multiply(x=60, y=w1361) -> (x*y=w1359:i32)
                          n1076 = Add(x=w1359, y=438) -> (x+y=w1356:i32)
                          n1077 = Bundle("y"=-1820, w1356) -> (w1355:cluster{"y":i32, i32})  [unwired: 1 in]
                          n1078 = property class="Bool (严格)"(reference=w1362, "Position"=w1355) -> ()  [unwired: 1 in, 2 out]
                        }
                      }
                      frame "R563X" {
                        # "1345"
                        n1079 = control-ref of="安装支架螺栓2拧紧确认"() -> (w1390:refnum<vi>)
                        n1080 = control-ref of="安装支架涂色标"() -> (w1389:refnum<vi>)
                        n1081 = control-ref of="安装支架螺栓1拧紧确认"() -> (w1391:refnum<vi>)
                        n1082 = control-ref of="控制器安装螺栓1拧紧确认"() -> (w1393:refnum<vi>)
                        n1083 = control-ref of="控制器安装螺栓2拧紧确认"() -> (w1392:refnum<vi>)
                        n1084 = control-ref of="安装弹性垫圈弹簧并按启动拍照"() -> (w1385:refnum<vi>)
                        n1085 = control-ref of="电机安装螺栓1扭矩确认"() -> (w1384:refnum<vi>)
                        n1086 = control-ref of="电机安装螺栓2扭矩确认"() -> (w1383:refnum<vi>)
                        n1087 = control-ref of="涂色标"() -> (w1381:refnum<vi>)
                        n1088 = control-ref of="安装扎带并取走工件"() -> (w1380:refnum<vi>)
                        n1089 = control-ref of="按启动按钮拍照确认"() -> (w1382:refnum<vi>)
                        n1090 = control-ref of="控制器支架螺栓2拧紧确认"() -> (w1387:refnum<vi>)
                        n1091 = control-ref of="控制器支架螺栓1拧紧确认"() -> (w1388:refnum<vi>)
                        n1092 = control-ref of="控制器支架螺栓3拧紧确认"() -> (w1386:refnum<vi>)
                        n1093 = control-ref of="控制器支架涂色标"() -> (w1379:refnum<vi>)
                        n1094 = Build Array(w1393, w1392, w1391, w1390, w1389) -> (w1396:refnum<vi>[])
                        n1095 = control-ref of="控制器支架螺栓5拧紧确认"() -> (w1374:refnum<vi>)
                        n1096 = control-ref of="控制器支架螺栓4拧紧确认"() -> (w1373:refnum<vi>)
                        n1097 = control-ref of="安装支架线卡扎带安装"() -> (w1372:refnum<vi>)
                        n1098 = for {
                          tunnel: w1396 -> [w1428] mode=indexing
                          i -> [w1427]
                          n1099 = Multiply(x=60, y=w1427) -> (x*y=w1422:i32)
                          n1100 = Add(x=438 ("y"), y=w1422) -> (x+y=w1424:i32)
                          n1101 = Bundle("y"=-1495, w1424) -> (w1423:cluster{"y":i32, i32})  [unwired: 1 in]
                          n1102 = property class="Bool (严格)"(reference=w1428, "Position"=w1423) -> ()  [unwired: 1 in, 2 out]
                        }
                        n1103 = Build Array(w1385, w1384, w1383, w1382, w1381, w1380) -> (w1394:refnum<vi>[])
                        n1104 = control-ref of="安装支架扎带安装"() -> (w1375:refnum<vi>)
                        n1105 = control-ref of="安装扎带和线卡并取走工件"() -> (w1376:refnum<vi>)
                        n1106 = control-ref of="控制器支架安装线卡扎带"() -> ()  [unwired: 1 out]
                        n1107 = control-ref of="控制器支架螺栓5拧紧确认"() -> (w1377:refnum<vi>)
                        n1108 = control-ref of="控制器支架螺栓4拧紧确认"() -> (w1378:refnum<vi>)
                        n1109 = for {
                          tunnel: w1394 -> [w1412] mode=indexing
                          i -> [w1411]
                          n1110 = Multiply(x=60, y=w1411) -> (x*y=w1409:i32)
                          n1111 = Add(x=w1409, y=438) -> (x+y=w1406:i32)
                          n1112 = Bundle("y"=-1145, w1406) -> (w1405:cluster{"y":i32, i32})  [unwired: 1 in]
                          n1113 = property class="Bool (严格)"(reference=w1412, "Position"=w1405) -> ()  [unwired: 1 in, 2 out]
                        }
                        n1114 = Build Array(w1388, w1387, w1386, w1379) -> (w1395:refnum<vi>[])
                        n1115 = Build Array(w1378, w1377, w1376, w1375, w1374, w1373, w1372) -> (w1371:refnum<vi>[])
                        n1116 = for {
                          tunnel: w1395 -> [w1420] mode=indexing
                          i -> [w1419]
                          n1117 = Multiply(x=60, y=w1419) -> (x*y=w1417:i32)
                          n1118 = Add(x=w1417, y=438) -> (x+y=w1414:i32)
                          n1119 = Bundle("y"=-1820, w1414) -> (w1413:cluster{"y":i32, i32})  [unwired: 1 in]
                          n1120 = property class="Bool (严格)"(reference=w1420, "Position"=w1413) -> ()  [unwired: 1 in, 2 out]
                        }
                        n1121 = for {
                          tunnel: w1371 -> [w1404] mode=indexing
                          i -> [w1403]
                          n1122 = Multiply(x=60, y=w1403) -> (x*y=w1401:i32)
                          n1123 = Add(x=w1401, y=438) -> (x+y=w1398:i32)
                          n1124 = Bundle("y"=-100, w1398) -> (w1397:cluster{"y":i32, i32})  [unwired: 1 in]
                          n1125 = property class="Bool (严格)"(reference=w1404, "Position"=w1397) -> ()  [unwired: 1 in, 2 out]
                        }
                      }
                    }
                  }
                  frame Enabled {
                  }
                }
              }
            }
          }
          event "更换产品": Value Change {
            n1126 = event-data() -> ()  [unwired: 1 in, 6 out]
            n1127 = control-ref of="控制器支架安装线卡扎带"() -> (w1459:refnum<vi>)
            n1128 = control-ref of="控制器支架螺栓5拧紧确认"() -> (w1461:refnum<vi>)
            n1129 = control-ref of="控制器支架涂色标"() -> (w1460:refnum<vi>)
            n1130 = control-ref of="控制器支架螺栓3拧紧确认"() -> (w1463:refnum<vi>)
            n1131 = control-ref of="控制器支架螺栓4拧紧确认"() -> (w1462:refnum<vi>)
            n1132 = control-ref of="控制器支架螺栓2拧紧确认"() -> (w1464:refnum<vi>)
            n1133 = control-ref of="控制器支架螺栓1拧紧确认"() -> (w1465:refnum<vi>)
            n1134 = control-ref of="安装支架螺栓4拧紧确认"() -> (w1449:refnum<vi>)
            n1135 = global read "Global.vi" "控制器支架"() -> (w1456:bool[])
            n1136 = control-ref of="安装支架线卡扎带安装"() -> (w1448:refnum<vi>)
            n1137 = control-ref of="安装支架螺栓2拧紧确认"() -> (w1451:refnum<vi>)
            n1138 = control-ref of="安装支架螺栓3拧紧确认"() -> (w1450:refnum<vi>)
            n1139 = control-ref of="安装支架涂色标"() -> (w1447:refnum<vi>)
            n1140 = control-ref of="安装扎带和线卡并取走工件"() -> (w1446:refnum<vi>)
            n1141 = control-ref of="控制器安装螺栓2拧紧确认"() -> (w1454:refnum<vi>)
            n1142 = control-ref of="安装支架螺栓1拧紧确认"() -> (w1452:refnum<vi>)
            n1143 = control-ref of="控制器安装螺栓3拧紧确认"() -> (w1453:refnum<vi>)
            n1144 = control-ref of="控制器安装螺栓1拧紧确认"() -> (w1455:refnum<vi>)
            n1145 = Build Array(w1465, w1464, w1463, w1462, w1461, w1460, w1459) -> (w1431:refnum<vi>[])
            n1146 = for "For循环" {
              tunnel: w1456 -> [w1499] mode=indexing
              tunnel: w1431 -> [w1498] mode=indexing
              shift-right: [w1496] -> _
              shift-left: 360 -> [w1497]
              tunnel: w1431 -> [w1495]
              i -> [w1494]
              n1147 = case shown="假" w1499 {
                tunnel: w1498 -> [w1501 w1503]
                tunnel: w1497 -> [w1502 w1508]
                tunnel: [w1502 w1505] -> w1496
                tunnel: w1495 -> [_ _]
                tunnel: w1494 -> [_ _]
                frame False {
                  n1148 = property class="Bool (严格)"(reference=w1501, "Top"=-100 ("位置:置顶")) -> ()  [unwired: 1 in, 2 out]
                }
                frame True {
                  n1149 = Add(x=w1508, y=50) -> (x+y=w1505:i32)
                  n1150 = Bundle(-1850, w1505) -> (w1506:cluster{i32, i32})  [unwired: 1 in]
                  n1151 = property class="Bool (严格)"(reference=w1503, "Position"=w1506) -> ()  [unwired: 1 in, 2 out]
                }
              }
            }
            n1152 = global read "Global.vi" "控制器安装支架"() -> (w1445:bool[])
            n1153 = Build Array(w1455, w1454, w1453, w1452, w1451, w1450, w1449, w1447, w1448, w1446) -> (w1444:refnum<vi>[])
            n1154 = for "For循环" {
              tunnel: w1445 -> [w1484] mode=indexing
              tunnel: w1444 -> [w1483] mode=indexing
              shift-right: [w1481] -> _
              shift-left: 360 -> [w1482]
              tunnel: w1444 -> [w1480]
              n1155 = case shown="真" w1484 {
                tunnel: w1483 -> [w1486 w1488]
                tunnel: w1482 -> [w1487 w1493]
                tunnel: [w1487 w1490] -> w1481
                tunnel: w1480 -> [_ _]
                frame False {
                  n1156 = property class="Bool (严格)"(reference=w1486, "Top"=-100 ("位置:置顶")) -> ()  [unwired: 1 in, 2 out]
                }
                frame True {
                  n1157 = Add(x=w1493, y=50) -> (x+y=w1490:i32)
                  n1158 = Bundle(-1510, w1490) -> (w1491:cluster{i32, i32})  [unwired: 1 in]
                  n1159 = property class="Bool (严格)"(reference=w1488, "Position"=w1491) -> ()  [unwired: 1 in, 2 out]
                }
              }
            }
            n1160 = control-ref of="电机安装螺栓1扭矩确认"() -> (w1441:refnum<vi>)
            n1161 = control-ref of="安装弹性垫圈弹簧并按启动拍照"() -> (w1442:refnum<vi>)
            n1162 = control-ref of="请拾取O型圈"() -> (w1430:refnum<vi>)
            n1163 = control-ref of="请拾取弹簧"() -> (w1429:refnum<vi>)
            n1164 = control-ref of="安装扎带并取走工件"() -> (w1435:refnum<vi>)
            n1165 = control-ref of="电机安装螺栓3扭矩确认"() -> (w1439:refnum<vi>)
            n1166 = control-ref of="电机安装螺栓2扭矩确认"() -> (w1440:refnum<vi>)
            n1167 = control-ref of="按启动按钮拍照确认"() -> (w1438:refnum<vi>)
            n1168 = control-ref of="安装支架扎带安装"() -> (w1436:refnum<vi>)
            n1169 = control-ref of="涂色标"() -> (w1437:refnum<vi>)
            n1170 = global read "Global.vi" "电机安装"() -> (w1433:bool[])
            n1171 = Build Array(w1429, w1430, w1442, w1441, w1440, w1439, w1438, w1437, w1436, w1435) -> (w1434:refnum<vi>[])
            n1172 = for "For循环" {
              tunnel: w1433 -> [w1470] mode=indexing
              tunnel: w1434 -> [w1469] mode=indexing
              shift-right: [w1467] -> _
              shift-left: 360 -> [w1468]
              tunnel: w1434 -> [w1466]
              n1173 = case shown="真" w1470 {
                tunnel: w1469 -> [w1472 w1474]
                tunnel: w1468 -> [w1473 w1479]
                tunnel: [w1473 w1476] -> w1467
                tunnel: w1466 -> [_ _]
                frame False {
                  n1174 = property class="Bool (严格)"(reference=w1472, "Top"=-100 ("位置:置顶")) -> ()  [unwired: 1 in, 2 out]
                }
                frame True {
                  n1175 = Add(x=w1479, y=50) -> (x+y=w1476:i32)
                  n1176 = Bundle(-1193, w1476) -> (w1477:cluster{i32, i32})  [unwired: 1 in]
                  n1177 = property class="Bool (严格)"(reference=w1474, "Position"=w1477) -> ()  [unwired: 1 in, 2 out]
                }
              }
            }
            "产品型号" <- w1457
          }
          event Panel Close {
            n1178 = event-data() -> ()  [unwired: 1 in, 4 out]
            n1179 = global write "Global.vi" "程序关闭"(TRUE ("程序关闭")) -> ()
          }
        }
        n1180 = case shown="真" w1151 {
          tunnel: w1150 -> [_ w1153]
          frame False {
          }
          frame True {
            n1181 = property on="更换布局" class="Str"("Val(Sgnl)"=w1153) -> ()  [unwired: 2 in, 2 out]
          }
        }
        n1182 = control-ref of="更换产品"() -> (w1148:refnum<vi>)
        n1183 = global write "Global.vi" "更换产品"(w1148) -> ()
        n1184 = global read "Global.vi" "程序关闭"() -> (w1149:bool)
      }
    }
  }
